vi "JL Dryer Tool.vi"() -> ()   [LabVIEW 2018]
uses:
  GExplorer Support/typedefs/GExplorer_Data_Cluster.ctl
  Common/LabVIEW GEA2 Toolkit/LabVIEW_GEA2_Toolkit.lvlibp/type defs/Data In.ctl
  JL Dryer Tool Support/type defs/ERD_Data_Loop_Control.ctl
  Common/LabVIEW GEA2 Toolkit/LabVIEW_GEA2_Toolkit.lvlibp/type defs/Data Type.ctl
  JL Dryer Tool Support/type defs/ERD_Loop_States_JL.ctl
  Common/LabVIEW GEA2 Toolkit/LabVIEW_GEA2_Toolkit.lvlibp/type defs/ERD Read Data In.ctl
  JL Dryer Tool Support/type defs/Error_Command.ctl
  JL Dryer Tool Support/type defs/DAQ_States.ctl
  JL Dryer Tool Support/type defs/Cont_Send_States.ctl
  <vilib>/DAQmx/write.llb/DAQmx Write (Analog 1D DBL NChan 1Samp).vi
  Common/LabVIEW GEA2 Toolkit/LabVIEW_GEA2_Toolkit.lvlibp/type defs/ERD Write Data In.ctl
  JL Dryer Tool Support/type defs/Flash_Results.ctl
  GEA2 Script/typedefs/Script Info.ctl
  JL Dryer Tool Support/type defs/GEA2_Control_Command.ctl
  JL Dryer Tool Support/type defs/ERD_Loop_Control_Command.ctl
  JL Dryer Tool Support/type defs/DAQ_Control_Command.ctl
  D:/Common/DLLs/GEA3/GeaCommunication.dll
  DLLs/GEA3/GeaCommunication.dll
  Common/LabVIEW GEA2 Toolkit/LabVIEW_GEA2_Toolkit.lvlibp/advanced/GEA2 Message Received Event Handler.vi
  Common/LabVIEW GEA2 Toolkit/LabVIEW_GEA2_Toolkit.lvlibp/advanced/GEA2 Message Sent Event Handler.vi
  Common/LabVIEW GEA2 Toolkit/LabVIEW_GEA2_Toolkit.lvlibp/type defs/Data Out.ctl
  Diagnostics Decode/Type Defs/Diag_FaultTableStatus.ctl
  <vilib>/DAQmx/create/channels.llb/DAQmx Create Channel (DI-Digital Input).vi
  <vilib>/DAQmx/create/channels.llb/DAQmx Create Channel (AO-Voltage-Basic).vi
  <vilib>/DAQmx/create/channels.llb/DAQmx Create Channel (DO-Digital Output).vi
  <vilib>/DAQmx/read.llb/DAQmx Read (Digital 1D Bool NChan 1Samp 1Line).vi
  <vilib>/DAQmx/write.llb/DAQmx Write (Digital 1D Bool NChan 1Samp 1Line).vi
  Common/LabVIEW GEA2 Toolkit/LabVIEW_GEA2_Toolkit.lvlibp/type defs/Source_Destination.ctl
  JL Dryer Tool Support/type defs/ERD_Graph.ctl
  JL Dryer Tool Support/type defs/ERD_Graph_All.ctl
  JL Dryer Tool Support/type defs/Select _Graph_JL.ctl
  JL Dryer Tool Support/type defs/Heat Control.ctl
  JL Dryer Tool Support/type defs/ERD_Always_Show_JL.ctl
  JL Dryer Tool Support/type defs/Programming.ctl
  JL Dryer Tool Support/type defs/Relay_Control.ctl
  JL Dryer Tool Support/type defs/Drum_Light_Control.ctl
  JL Dryer Tool Support/UTL_JL Scaling Factor Folder/Controls/ENUM_JL Scaling Factor_.ctl
  JL Dryer Tool Support/type defs/Cycle Control.ctl
  <vilib>/Platform/fileVersionInfo.llb/FileVersionInformation.ctl
  JL Dryer Tool Support/type defs/Choose_ERD_List.ctl
  Automation/Product Specific/Clothes Care/Justice League/Product Testcode/Diagnostics/TypeDefs/Centauro Diagnostic V3 SnapShot.ctl
  Diagnostics Decode/Type Defs/Diag_FaultSeqEntry.ctl
  Diagnostics Decode/Type Defs/Diag_EntityManifestType.ctl
  Diagnostics Decode/Type Defs/Diag_FaultTableEntry.ctl
  JL Dryer Tool Support/type defs/JL_Diagnost V3 Cycle History.ctl
panel:
  out "Temp ADC":T1
  in  "Read Parametric":bool=TRUE
  in  "Board Index 2":u8 max=0 step=1
  in  "Data ON":bool=TRUE
  out "ERD_Always Show":T2
  in  "Stop":bool
  in  "Reset":bool
  in  "UI Launch":bool
  in  "Tab Control":T3(tab)
  out "Boot Loader Version":T4
  out "UI Version":T5
  out "Version":T6
  in  "Flash Latest":bool
  in  "Filter Data":bool=TRUE
  in  "Start Send":bool
  in  "Ignore this CMD":string
  in  "Msg Rate (ms)":u32=1000 min=50 step=50
  out "Personality Set":u8
  in  "?":u8
  in  "Set Personality":bool
  in  "Programming":T7={"Program"=FALSE, "File Path"=path "", "Program Ind"=FALSE, "Reset Board"=FALSE, "Enter Bootloader"=FALSE, "Result"=9} {"Result" items=["ImageRejected", "BoardNotFound", "UnableToGetGeaConfiguration", "WriteToFlashNotAllowed", "ImageDownloadedSuccessfully", "ImagePresent", "WriteToFlashFailed", "EraseFailed", "CrcFailed", ""]}
  out "CSV File Log Path":path=path "C:/Users/502129737/Desktop/1"
  in  "Clear":bool
  out "GEA2 Log":string
  in  "Board Index":u8 max=10 step=1
  out "Board ID":string="0"
  in  "GEA2 Send":T9={"Source"=228, "Destination"=36, "Command"=0, "Message"=""} {"Command" format="%02x"; "Destination" format="%02x"; "Source" format="%02x"}
  in  "Send Button":bool
  in  "GEA2 Log Length":i32=100000
  in  "Save Log":bool
  in  "#ERDs per message":i32=20
  out "FileVersionInfo":T10
  out "LabView/Version Number":string
  in  "Tool Version":bool=TRUE
  in  "GEA Inputs":T11={"Source"=229, "Destination"=36} {"Destination" format="%.0x"; "Source" format="%.0x"}
  in  "Read ERD List":T12[](array[typedef])=[{"ERD Number"=0, "Data Type"=enum."string"}] {"ERD Number" format="%.0x"}
  out "Read ERD Data Out":cluster{"ERD Number":u16, "Data":string}[](array[cluster]) {"ERD Number" format="%.0x"}
  in  "Read ERD":bool
  in  "Write ERD":bool
  in  "Write ERD List":T14(array[cluster])=[{"ERD Number"=0, "Data Type"=enum."string", "Data"=""}] {"ERD Number" format="%.0x"}
  in  "ERD Graphing ON":bool
  out "ERD Graph  Ind":T15
  in  "ERD Graph Cntrl":T16={"ERD 3"={"ERD #"=61463, "Data Type"=enum."uint16_t", "Scaler"=1}, "ERD 2"={"ERD #"=61461, "Data Type"=enum."uint16_t", "Scaler"=1}, "ERD 1"={"ERD #"=61462, "Data Type"=enum."uint16_t", "Scaler"=1}} {"ERD 1"."Scaler" min=1; "ERD 1"."ERD #" format="%.0x"; "ERD 2"."Scaler" min=1; "ERD 2"."ERD #" format="%.0x"; "ERD 3"."Scaler" min=1; "ERD 3"."ERD #" format="%.0x"}
  in  "Graphing ON":bool=TRUE
  in  "Select Graph":T18
  out "Outlet Thermistor":u16(graph)
  out "Filtered Moisture":u16(graph)
  out "Raw Moisture":u16(graph)
  out "All Loads":u16[][](graph)
  out "ERD 1":dbl(graph)
  out "ERD 2":dbl(graph)
  out "Inlet Thermistor":u16(graph)
  out "ERD 3":dbl(graph)
  in  "Get Faults":bool
  in  "Clear Fault Table Buffer":bool
  in  "Clear Fault Seq Buffer":bool
  out "Fault Sequence Entries":T19[](array[typedef])
  out "Fault Seq Status":T20
  out "Fault Table Entries":T21[](array[typedef])
  out "Fault Table Status":T20
  out "Diagnostic Entity Manifest":T22
  out "Major Version":u8
  out "Minor Version":u8
  out "Fault Set?":bool
  in  "Filter by Count":bool=TRUE
  out "Centauro Fault Snapshot":T23
  in  "Drum Light":T24={"Drum Light ON"=FALSE, "Drum Light OFF"=FALSE, "On Time (s)"=5.0} {"On Time (s)" min=0.0 max=3600.0}
  in  "Relay Control":T25
  in  "LED Control":T26
  in  "Cycle Control":T27
  in  "Enable CC Mode":bool
  in  "Completed Cycles":u16
  in  "Requested Cycles":u16
  in  "TimeBetween Cycles":u32
  in  "Enabled":u8
  in  "ERD Spam GEA Inputs":T11={"Source"=229, "Destination"=36} {"Destination" format="%.0x"; "Source" format="%.0x"}
  in  "Normal Temp V":bool=TRUE
  in  "Manual Inlet":dbl format="%#_13g"
  in  "Manual Outlet":dbl format="%#_13g"
  out "Heat Control":T28
  in  "Init/Scale":T29=enum."Scale Voltage"
  in  "Scalling":T30={"Low  "=1531.0, " High"=6859.0, "Actual Low"=1.0, "Actual High"=4.9}
  in  "Desired FilteredMoisture":dbl=2400.0 min=1000.0 max=6300.0 step=5.0
  out "Drum":bool
  out "Centrifugal Switch":bool caption="Cent SW"
  out "Drum Direction":string
  in  "CentSWControl":bool
  in  "CentSWControlType":bool=TRUE
  out "Steam":bool
  out "Drum Light":bool
  out "Outer Coil":bool
  out "Inner/Gas Coil":bool
  in  "Dither (V)":dbl=0.05 min=0.0 max=1.0 step=0.001 format="%_3g"
  in  "Outlet Therm (F)":dbl(knob)=75.0 min=49.0 max=201.0 step=1.0 scale=50.0..200.0
  in  "Inlet Therm (F)":u16(knob)=75 min=49 max=501 step=1 scale=50.0..500.0
  in  "Moisture (V)":dbl(slide)=1.945 min=0.0 max=5.0 step=0.0001 scale=0.0..5.0 scale format="%#.2f"
  in  "AC Power":bool=TRUE
  in  "Door Status":bool=TRUE
  in  "Start Signal":bool
  out "DAQ Status":string
  in  "Turn On DAQ":bool
  out "DAQ On?":bool
  out "Inlet Voltage":dbl
  out "Outlet Voltage":dbl
  in  "Model":enum16{"Estar Centauro", "GFL"}(ring)
  out "Dampness State":string
  out "Sensor Dry Status":string
  in  "Get Cycle Data":bool
  out "Cycle History Status":T20
  in  "Filter by Status Count":bool=TRUE
  out "JL Cycle History":T31
  in  "Script Log Path":path
  in  "Run Script":bool
  out "Script Pass/Fail?":bool
  out "Script Report Text":string
  in  "stop script":bool
  in  "Script Path":path
  out "Script Info":T32 {"Overall Script File Progress" scale=0.0..1.0; "Elapsed time (s)" format="%#.1f"; "Current Script Progress" scale=0.0..1.0}
  out "Script Error Out":errorcluster
  in  "ERD Read List":T33(array[cluster])=[{"Boolean"=TRUE, "ERD Number"=49, "ERD Name"="Build Number", "Data Type"=enum."uint32_t"}, {"Boolean"=TRUE, "ERD Number"=127, "ERD Name"="Build Hash", "Data Type"=enum."string"}, {"Boolean"=TRUE, "ERD Number"=61467, "ERD Name"="Machine State", "Data Type"=enum."uint8_t"}, {"Boolean"=TRUE, "ERD Number"=61457, "ERD Name"="Relay Status", "Data Type"=enum."string"}, {"Boolean"=TRUE, "ERD Number"=61459, "ERD Name"="Door Switch State", "Data Type"=enum."string"}, {"Boolean"=TRUE, "ERD Number"=61460, "ERD Name"="Door Latch State", "Data Type"=enum."string"}, {"Boolean"=TRUE, "ERD Number"=61461, "ERD Name"="Inlet Thermistor", "Data Type"=enum."uint16_t"}, {"Boolean"=TRUE, "ERD Number"=61462, "ERD Name"="Outlet Thermistor", "Data Type"=enum."uint16_t"}, {"Boolean"=TRUE, "ERD Number"=61468, "ERD Name"="Control Lock State", "Data Type"=enum."string"}, {"Boolean"=TRUE, "ERD Number"=61483, "ERD Name"="Signal Volume", "Data Type"=enum."string"}, {"Boolean"=TRUE, "ERD Number"=61582, "ERD Name"="Drum Light", "Data Type"=enum."string"}, {"Boolean"=TRUE, "ERD Number"=61478, "ERD Name"="Delay Time", "Data Type"=enum."string"}, {"Boolean"=TRUE, "ERD Number"=8275, "ERD Name"="Ext. Tumble", "Data Type"=enum."string"}, {"Boolean"=TRUE, "ERD Number"=8272, "ERD Name"="Temp Level", "Data Type"=enum."string"}, {"Boolean"=TRUE, "ERD Number"=8269, "ERD Name"="Dryness Level", "Data Type"=enum."string"}, {"Boolean"=TRUE, "ERD Number"=8262, "ERD Name"="eDry", "Data Type"=enum."string"}, {"Boolean"=TRUE, "ERD Number"=61495, "ERD Name"="Time Level", "Data Type"=enum."string"}, {"Boolean"=TRUE, "ERD Number"=8266, "ERD Name"="Damp Alert", "Data Type"=enum."string"}, {"Boolean"=TRUE, "ERD Number"=61501, "ERD Name"="Detangle", "Data Type"=enum."string"}, {"Boolean"=TRUE, "ERD Number"=61510, "ERD Name"="MyCycle", "Data Type"=enum."string"}, {"Boolean"=TRUE, "ERD Number"=61594, "ERD Name"="Cycle Engine State", "Data Type"=enum."string"}, {"Boolean"=TRUE, "ERD Number"=61597, "ERD Name"="Cycle Selected", "Data Type"=enum."string"}, {"Boolean"=TRUE, "ERD Number"=61443, "ERD Name"="Tune ID", "Data Type"=enum."string"}, {"Boolean"=TRUE, "ERD Number"=61503, "ERD Name"="Delay Option", "Data Type"=enum."string"}, {"Boolean"=TRUE, "ERD Number"=61619, "ERD Name"="Restriction Detection Status", "Data Type"=enum."string"}, {"Boolean"=TRUE, "ERD Number"=61618, "ERD Name"="Vent Restriction", "Data Type"=enum."string"}, {"Boolean"=TRUE, "ERD Number"=61611, "ERD Name"="Load Size By Contact", "Data Type"=enum."string"}, {"Boolean"=TRUE, "ERD Number"=61613, "ERD Name"="Load Size by Temp", "Data Type"=enum."string"}, {"Boolean"=TRUE, "ERD Number"=61615, "ERD Name"="LoadSizeByAggregation", "Data Type"=enum."string"}, {"Boolean"=TRUE, "ERD Number"=61605, "ERD Name"="Sensor Dry Status", "Data Type"=enum."string"}, {"Boolean"=TRUE, "ERD Number"=61626, "ERD Name"="Check Dampness State", "Data Type"=enum."string"}, {"Boolean"=TRUE, "ERD Number"=61624, "ERD Name"="MoistureSensorRawAdcFromMc", "Data Type"=enum."string"}, {"Boolean"=TRUE, "ERD Number"=62242, "ERD Name"="SmoothMoistureReading", "Data Type"=enum."string"}, {"Boolean"=TRUE, "ERD Number"=61463, "ERD Name"="Filtered Moisture", "Data Type"=enum."string"}, {"Boolean"=TRUE, "ERD Number"=61608, "ERD Name"="TargetMoistureVoltage", "Data Type"=enum."string"}, {"Boolean"=TRUE, "ERD Number"=61609, "ERD Name"="TargetMoistureVoltageReached", "Data Type"=enum."string"}, {"Boolean"=TRUE, "ERD Number"=61719, "ERD Name"="MaxFilteredMoistureVoltageDuringASensingCycle", "Data Type"=enum."string"}, {"Boolean"=TRUE, "ERD Number"=61555, "ERD Name"="TrimmerBothCoilInhibitRequest", "Data Type"=enum."string"}, {"Boolean"=TRUE, "ERD Number"=61567, "ERD Name"="TrimmerInhibitRelay1", "Data Type"=enum."string"}, {"Boolean"=TRUE, "ERD Number"=61568, "ERD Name"="TrimmerInhibitRelay2", "Data Type"=enum."string"}, {"Boolean"=TRUE, "ERD Number"=61549, "ERD Name"="HeatControlParametricData", "Data Type"=enum."string"}, {"Boolean"=TRUE, "ERD Number"=61610, "ERD Name"="EOC Reason", "Data Type"=enum."string"}, {"Boolean"=TRUE, "ERD Number"=61600, "ERD Name"="Heat Control Request", "Data Type"=enum."string"}, {"Boolean"=TRUE, "ERD Number"=61677, "ERD Name"="CoolDownStepStatus", "Data Type"=enum."string"}, {"Boolean"=TRUE, "ERD Number"=61554, "ERD Name"="OverTempHeaterInhibitRequest", "Data Type"=enum."string"}, {"Boolean"=TRUE, "ERD Number"=61565, "ERD Name"="EcoDryInhibitRelay1", "Data Type"=enum."string"}, {"Boolean"=TRUE, "ERD Number"=61566, "ERD Name"="EcoDryInhibitRelay2", "Data Type"=enum."string"}, {"Boolean"=TRUE, "ERD Number"=61743, "ERD Name"="ReverseDrumInhibitRelay1", "Data Type"=enum."string"}, {"Boolean"=TRUE, "ERD Number"=61744, "ERD Name"="ReverseDrumInhibitRelay2", "Data Type"=enum."string"}, {"Boolean"=TRUE, "ERD Number"=61556, "ERD Name"="NormalHeatControlMethodStatus", "Data Type"=enum."string"}, {"Boolean"=TRUE, "ERD Number"=61557, "ERD Name"="FallbackHeatControlMethodStatus", "Data Type"=enum."string"}, {"Boolean"=TRUE, "ERD Number"=61479, "ERD Name"="Remaining Cycle Time", "Data Type"=enum."string"}, {"Boolean"=TRUE, "ERD Number"=61698, "ERD Name"="InitialHeatingCycleTimeSeconds", "Data Type"=enum."string"}, {"Boolean"=TRUE, "ERD Number"=62214, "ERD Name"="InletTemperatureRawAdc\n", "Data Type"=enum."string"}, {"Boolean"=TRUE, "ERD Number"=62215, "ERD Name"="OutletTemperatureRawAdc", "Data Type"=enum."string"}, {"Boolean"=TRUE, "ERD Number"=61607, "ERD Name"="SensingCycleTotalDryingTimeSeconds", "Data Type"=enum."string"}, {"Boolean"=TRUE, "ERD Number"=61563, "ERD Name"="TimedCycleTotalDryingTimeSeconds", "Data Type"=enum."string"}, {"Boolean"=TRUE, "ERD Number"=61628, "ERD Name"="TimeToReachTargetVoltageSeconds", "Data Type"=enum."string"}, {"Boolean"=TRUE, "ERD Number"=61617, "ERD Name"="Dry Load Detection", "Data Type"=enum."string"}, {"Boolean"=TRUE, "ERD Number"=63510, "ERD Name"="Sensor DryTemp Multiplier 100", "Data Type"=enum."string"}, {"Boolean"=TRUE, "ERD Number"=61728, "ERD Name"="Erd_EcoDrySensorDryProfileSelectorStatus", "Data Type"=enum."string"}, {"Boolean"=TRUE, "ERD Number"=61729, "ERD Name"="Erd_EcoDrySensorDryProfileSelectorResultmeInSeconds", "Data Type"=enum."string"}, {"Boolean"=TRUE, "ERD Number"=61736, "ERD Name"="Erd_EcoDryControllerStatus", "Data Type"=enum."string"}, {"Boolean"=TRUE, "ERD Number"=61737, "ERD Name"="Erd_EcoDryRelay1TimerData", "Data Type"=enum."string"}, {"Boolean"=TRUE, "ERD Number"=61738, "ERD Name"="Erd_EcoDryRelay2TimerData", "Data Type"=enum."string"}, {"Boolean"=TRUE, "ERD Number"=61739, "ERD Name"="Erd_EcoDryStage2TransitionTimeInSeconds", "Data Type"=enum."string"}, {"Boolean"=TRUE, "ERD Number"=8193, "ERD Name"="Erd_MachineSubCycle", "Data Type"=enum."string"}, {"Boolean"=TRUE, "ERD Number"=61606, "ERD Name"="Erd_ElapsedCycleTimeSeconds2TransitionTimeInSeconds", "Data Type"=enum."string"}, {"Boolean"=TRUE, "ERD Number"=63489, "ERD Name"="SensorDryDampSmallRestrictionSmallLoad\natus", "Data Type"=enum."string"}] {"ERD Number" format="%.0x"}
  in  "Load ERD List":T34=enum."QA ERDs"
  out "Error Out":errorcluster
  in  "Error In":errorcluster
  # "The higher this number is the less reliable the bus becomes.\nLower will increase the delay for the ERD Array to populate.\nNo greater than 30 per msg is recommended. (crashing can occur)"
  # "Software Version"
  # "Critical Version"
  # "Non-Critical"
  # "Software Version"
  # "Critical Version"
  # "Non-Critical"
  # "XML Crit Ver"
  # "XML Non-Crit"
  # "Build Number"
  # "Build Hash"
  # "Personality"
  # "ERD_Graph_All.ctlERD_Graph_All.ctlMust input av valid ERD# and Data Type DO NOT Leave Blank If no scaler use value of 01"
  # "This controls destination of ERD Spam.\nYou should never change source unless\nyou want to see the spam in the GEA log."
  # "Continuous cycle Config"
  # "Filtered Moisture"
  # "Voltage (DAQ)"
  # "Measured Range"
  # "Centrifugal Switch"
  # "On"
  # "Normal"
  # "Off"
  # "Manual"
  # "Insert all New ERDs above F801..ensure this is the last ERD in the list"
  # "Contact:\n\nTerrance Bradford\nTerrance.Bradford@geappliances.com"
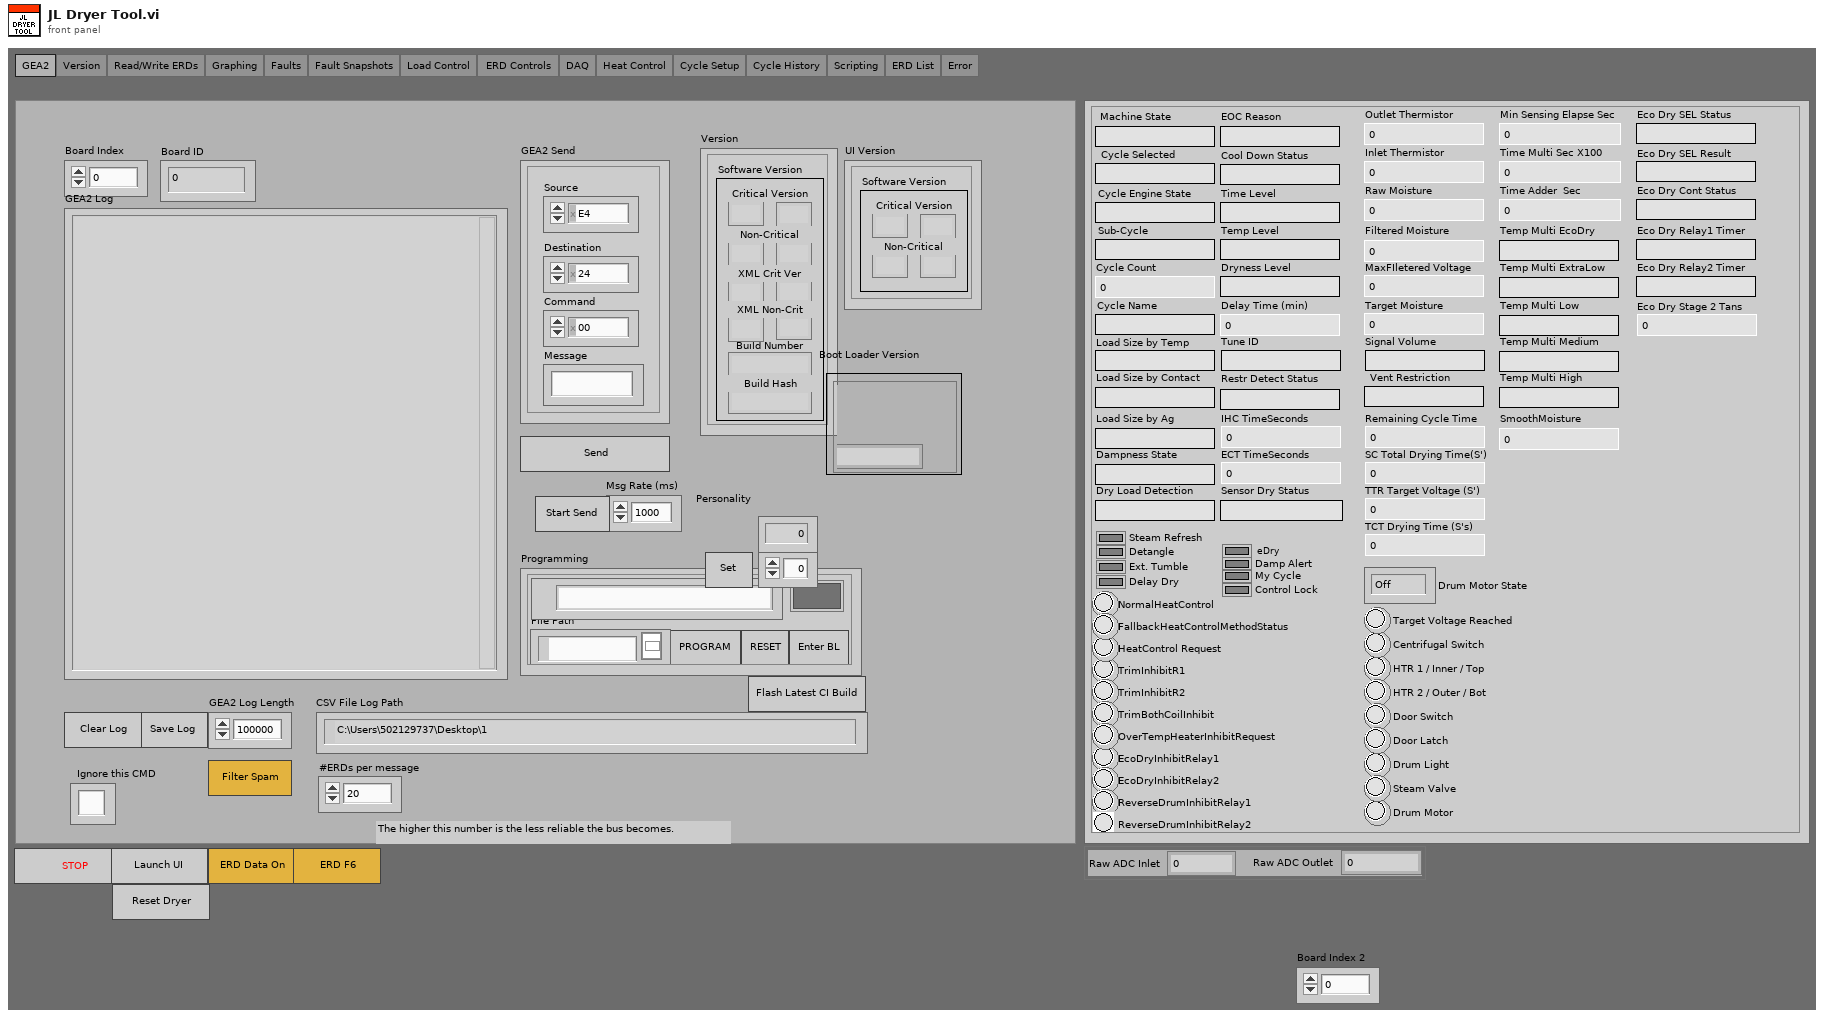
[diagram p1: front panel]
types:
  T1 = cluster{"Raw ADC Outlet":u16, "Raw ADC Inlet":u16}
  T2 = typedef "ERD_Always_Show_JL.ctl" = cluster{"Inlet Thermistor":u16, "Machine State":string, "Filtered Moisture":u16, "Cycle Selected":string, "HTR 1 / Inner / Top":bool, "HTR 2 / Outer / Bot":bool, "Door Switch":bool, "Drum Light":bool, "Cycle Engine State":string, "Centrifugal Switch":bool, "Drum Motor":bool, "Cycle Count":u32, "Ext. Tumble":bool, "eDry":bool, "Temp Level":string, "Dryness Level":string, "Time Level":string, "Delay Time (min)":u16, "Steam Refresh":bool, "Damp Alert":bool, "Sub-Cycle":string, "Outlet Thermistor":u16, "Target Moisture":u16, "Remaining Cycle Time":u32, "Raw Moisture":u16, "Cycle Name":string, "My Cycle":bool, "Delay Dry":bool, "Detangle":bool, "Control Lock":bool, "Steam Valve":bool, "Door Latch":bool, "Signal Volume":string, "Tune ID":string, "Restr Detect Status":string, "Vent Restriction":string, "Load Size by Contact":string, "Load Size by Temp":string, "EOC Reason":string, "Sensor Dry Status":string, "Dampness State":string, "Target Voltage Reached":bool, "TrimInhibitR1":bool, "TrimInhibitR2":bool, "TrimBothCoilInhibit":bool, "NormalHeatControl":bool, "HeatControl Request":bool, "Cool Down Status":string, "EcoDryInhibitRelay1":bool, "EcoDryInhibitRelay2":bool, "ReverseDrumInhibitRelay1":bool, "ReverseDrumInhibitRelay2":bool, "OverTempHeaterInhibitRequest":bool, "FallbackHeatControlMethodStatus":bool, "IHC TimeSeconds":u32, "ECT TimeSeconds ":u32, "SC Total Drying Time(S')":u32, "TTR Target Voltage (S')":u32, "TCT Drying Time (S's)":u32, "Drum Motor State":enum16{"Off", "Cw", "Ccw", "Max"}, "Load Size by Ag":string, "MaxFIletered Voltage":u16, "Dry Load Detection":string, "Min Sensing Elapse Sec":u32, "Time Multi Sec X100":u32, "Time Adder  Sec":u32, "Temp Multi EcoDry":string, "Temp Multi ExtraLow":string, "Temp Multi Low ":string, "Temp Multi Medium":string, "Temp Multi High":string, "SmoothMoisture":u16, "Eco Dry SEL Status":string, "Eco Dry SEL Result":string, "Eco Dry Cont Status":string, "Eco Dry Relay1 Timer":string, "Eco Dry Relay2 Timer ":string, "Eco Dry Stage 2 Tans ":u32}
  T3 = enum32{"GEA2", "Version", "Read/Write ERDs", "Graphing", "Faults", "Fault Snapshots", "Load Control", "ERD Controls ", "DAQ", "Heat Control", "Cycle Setup", "Cycle History", "Scripting", "ERD List", "Error"}
  T4 = cluster{"UI BL Version":string, "MC BL Version":string}
  T5 = cluster{"Critical Major":string, "Critical Minor":string, "Non-Critical Minor":string, "Non-Critical Major":string}
  T6 = cluster{"Critical Major":string, "Critical Minor":string, "Non-Critical Minor":string, "Non-Critical Major":string, "XML Crit Minor":string, "XMLCrit Major":string, "Build Number":string, "XML Non-crit Minor":string, "Xml Non-crit Major":string, "Build Hash":string}
  T7 = typedef "Programming.ctl" = cluster{"Program":bool, "File Path":path, "Program Ind":bool, "Reset Board":bool, "Enter Bootloader":bool, "Result":T8}
  T8 = typedef "Flash_Results.ctl" = i32
  T9 = typedef "LabVIEW_GEA2_Toolkit.lvlibp/Data In.ctl" = cluster{"Source":u8, "Destination":u8, "Command":u8, "Message":string}
  T10 = typedef "FileVersionInformation.ctl" = cluster{"FileVersion":string, "ProductName":string, "InternalName":string, "CompanyName":string, "LegalCopyright":string, "FileDescription":string}
  T11 = typedef "LabVIEW_GEA2_Toolkit.lvlibp/Source_Destination.ctl" = cluster{"Source":u8, "Destination":u8}
  T12 = typedef "LabVIEW_GEA2_Toolkit.lvlibp/ERD Read Data In.ctl" = cluster{"ERD Number":u16, "Data Type":T13}
  T13 = typedef "LabVIEW_GEA2_Toolkit.lvlibp/Data Type.ctl" = enum16{"string", "boolean", "uint8_t", "uint16_t", "uint32_t", "uint64_t", "int8_t", "int16_t", "int32_t", "int64_t"}
  T14 = cluster{"ERD Number":u16, "Data Type":T13, "Data":string}[]
  T15 = cluster{"ERD Value 1":dbl, "ERD Value 2":dbl, "ERD Value 3":dbl}
  T16 = typedef "ERD_Graph_All.ctl" = cluster{"ERD 3":T17, "ERD 2":T17, "ERD 1":T17}
  T17 = typedef "ERD_Graph.ctl" = cluster{"ERD #":u16, "Data Type":T13, "Scaler":u32}
  T18 = typedef "Select _Graph_JL.ctl" = enum16{"All Loads", "Inlet Thermistor", "Outlet Thermistor", "Raw Moisture", "Filtered Moisture", "ERD 1", "ERD 2", "ERD 3"}
  T19 = typedef "Diag_FaultSeqEntry.ctl" = cluster{"Cycle #":u32, "Time":u32, "F Code":string, "F Active":bool}
  T20 = typedef "Diag_FaultTableStatus.ctl" = cluster{"Cur Index":u16, "Count":u16, "Ov Cnt":u16}
  T21 = typedef "Diag_FaultTableEntry.ctl" = cluster{"Cycle #":u32, "Time":u32, "F Code":string, "F Count":u16, "F Active":bool}
  T22 = typedef "Diag_EntityManifestType.ctl" = cluster{"ID":u8, "Data Ver Maj":u8, "Data Ver Min":u8, "Fault Table?":bool, "Fault Table Snap?":bool, "Fault Seq?":bool, "Fault Seq Snap?":bool, "Cycle History Seq?":bool, "Fault Table Entry Count":u16, "Fault Seq Entry Count":u16, "Cycle History Entry Count":u16, "Cycle Count":u32, "Entity Run Time (Min)":u32}
  T23 = typedef "Centauro Diagnostic V3 SnapShot.ctl" = string[][]
  T24 = typedef "Drum_Light_Control.ctl" = cluster{"Drum Light ON":bool, "Drum Light OFF":bool, "On Time (s)":dbl}
  T25 = typedef "Relay_Control.ctl" = cluster{"Drum Motor":bool, "HTR 2 / Outer / Bot":bool, "Steam Valve":bool, "Relays ON":bool, "Relays OFF":bool, "HTR 1 / Inner / Top":bool}
  T26 = cluster{"ALL LEDs ON":bool, "ALL LEDs OFF":bool, "Reset LEDs":bool}
  T27 = typedef "Cycle Control.ctl" = cluster{"Start Cycle":bool, "Cycle Selection":u8, "Stop Cycle":bool, "Pause Cycle":bool, "Resume Cycle":bool, "Select Cycle":bool}
  T28 = typedef "Heat Control.ctl" = cluster{"Htr1 InletLowLim":string, "Htr1 InletUpLim":string, "Htr1 OutletLowLim":string, "Htr1 OutletUpLim":string, "Htr1 FallBackON(s)":string, "Htr1 FallBackOFF(s)":string, "Htr1":bool, "Htr2 InletLowLim":string, "Htr2 InletUpLim":string, "Htr2 OutletLowLim":string, "Htr2 OutletUpLim":string, "Htr2 FallBackON(s)":string, "Htr2 FallBackOFF(s)":string, "Htr2":bool}
  T29 = typedef "ENUM_JL Scaling Factor_.ctl" = enum16{"Init", "Scale Voltage", "Flush Slope"}
  T30 = cluster{"Low  ":dbl, " High":dbl, "Actual Low":dbl, "Actual High":dbl}
  T31 = typedef "JL_Diagnost V3 Cycle History.ctl" = string[][]
  T32 = typedef "Script Info.ctl" = cluster{"Overall Script File Progress":dbl, "Current Script Progress":dbl, "Script":string, "Test":string, "Elapsed time (s)":dbl, "Done?":bool}
  T33 = cluster{"Boolean":bool, "ERD Number":u16, "ERD Name":string, "Data Type":enum16{"string", "boolean", "uint8_t", "uint16_t", "uint32_t", "uint64_t", "int8_t", "int16_t", "int32_t", "int64_t"}}[]
  T34 = typedef "Choose_ERD_List.ctl" = enum16{"Base ERDs", "QA ERDs", "MABE ERD List", "EcoDry Evaluation ERD List", "ClothDampnessCheck ERD List"}
  T35 = typedef "Cont_Send_States.ctl" = enum16{"Run", "Shutdown"}
  T36 = typedef "DAQ_States.ctl" = enum16{"Wait for Init", "Rename Devices", "Verify Hardware", "Initialize", "Run", "Shutdown", "Exit"}
  T37 = typedef "ERD_Data_Loop_Control.ctl" = cluster{"Data":variant, "State":T38}
  T38 = typedef "ERD_Loop_States_JL.ctl" = enum16{"Init", "Build ERD Read List", "Read ERDs", "Get Version", "Check Load Size", "Update UI", "Update Graphs", "Read Faults", "Log Data", "Pause", "Shutdown"}
  T39 = typedef "Error_Command.ctl" = enum16{"Initialize", "Handle Errors", "Report Errors"}
  T40 = typedef "GExplorer_Data_Cluster.ctl" = cluster{"Data":variant, "State":enum16{"Add to Log", "Clear", "Shutdown"}}
  T41 = enum8{"Enabled", "Disabled", "Disabled and Grayed Out"}
  T42 = typedef "LabVIEW_GEA2_Toolkit.lvlibp/ERD Write Data In.ctl" = cluster{"ERD Number":u16, "Data Type":T13, "Data":string}
  T43 = enum16{"UI Application APL", "UI Parametric APL", "MC APL"}
  T44 = typedef "GEA2_Control_Command.ctl" = enum16{"Initialize", "Shutdown"}
  T45 = typedef "ERD_Loop_Control_Command.ctl" = enum16{"Initialize", "Shutdown"}
  T46 = typedef "DAQ_Control_Command.ctl" = enum16{"Initialize", "Shutdown", "Exit"}
  T47 = typedef "LabVIEW_GEA2_Toolkit.lvlibp/Data Out.ctl" = cluster{"Source":u8, "Destination":u8, "Command":u8, "Length":u8, "CRC":u16, "Message":string}
  T48 = typedef "LabVIEW_GEA2_Toolkit.lvlibp/ERD Read Data Out.ctl" = cluster{"ERD Number":u16, "Data":string}
  T49 = typedef "All_Bundled_Data_JL.ctl" = cluster{"Version":T50, "ERD_Always Show":T2, "Personality Set":u8, "CSV File String Arrays":T51, "Fault Table Array ":T52, "Heat Control":T28, "Temp ADC":cluster{"Raw ADC Outlet":u16, "Raw ADC Inlet":u16}, "UI Version":cluster{"Critical Major":string, "Critical Minor":string, "Non-Critical Minor":string, "Non-Critical Major":string}, "Boot Loader Version":cluster{"UI BL Version":string, "MC BL Version":string}}
  T50 = typedef "Version.ctl" = cluster{"Critical Major":string, "Critical Minor":string, "Non-Critical Minor":string, "Non-Critical Major":string, "XML Crit Minor":string, "XMLCrit Major":string, "Build Number":string, "XML Non-crit Minor":string, "Xml Non-crit Major":string, "Build Hash":string}
  T51 = typedef "CSV_File_String_Arrays.ctl" = cluster{"ERD Number Array":string[], "ERD Name Array":string[], "ERD Converted String Data":string[]}
  T52 = typedef "Fault Table Array.ctl" = T53[]
  T53 = typedef "Fault_Table_Info.ctl" = cluster{"Cycle Count":u32, " Runtime (min) ":u32, "Fault Status":string, "Fault ID":string, "Fault Count":u16}
  T54 = typedef "F6_ERD_Control.ctl" = cluster{"EcoDryEnabledFlag":string, "KeyCycleId":u8, "CycleType":string, "Time LVL option 5":u32, "Time LVL option 4":u32, "Time LVL option _3":u32, "Time LVL option _2":u32, "Time LVL option _1":u32, "Time LVL option _0":u32, "CoolDownTimeInSeconds":u32, "TimeAdjustTimeCycleMinimumTimeInSeconds":u32, "TimeAdjustTimeCycleMaximumTimeInSeconds":u32, "TimeAdjustTimeCycleStandardAdjustTimeInSeconds":u32, "TimeAdjustTimeCycleSlewAdjustTimeInSeconds":u32, "ExtendedTumbleTimeInSeconds":u32, "SanitizeMaxDryTimeInSeconds":u32, "TemperatureDefault Level":u8, "Temperature ecoDryDefualtLevel":u8, "DrynessDefault Level":u8, "DrynessDefault ecoDryDefualtLevel":u8, "TimeAdjust defaultLevel":u8, "TimeAdjust ecoDryDefualtLevel":u8, "TimeLevelDefault Level":u8, "TimeLevelDefault Eco Dry":u8, "EStarSensorDry Default Level":u8, "EStarSensorDry ecoDryDefaultLevel":u8, "EcoDryDefault Level":u8, "EcoDryDefault EcoDryDefaultLevel ":u8, "ExtendedTumble Default Level":u8, "ExtendedTumble  EcoDryDefaultLevel":u8, "Sanitize Default Level":u8, "Sanitize ecoDryDefualtLevel":u8, "MyCycleDefault Level":u8, "MyCycleDefault ecoDryDefualtLevel":u8, "StartPause Default Level":u8, "StartPause ecoDryDefualtLevel":u8, "Power Default Level":u8, "Power ecoDryDefualtLevel":u8, "KeyVolume Default Level":u8, "KeyVolume ecoDryDefualtLevel":u8, "AlertVolume Default Level":u8, "AlertVolume ecoDryDefualtLevel":u8, "ControlLock Default Level":u8, "ControlLock EecoDryDefualtLevel":u8, "HeatControlRelay1EcoDryParametricDataEntry\nHeatControlTemperatureLimit_InletLower":u16, "HeatControlRelay1EcoDryParametricDataEntry\nHeatControlTemperatureLimit_InletUpper":u16, "HeatControlRelay1EcoDryParametricDataEntry\nHeatControlTemperatureLimit_OutletLower":u16, "HeatControlRelay1EcoDryParametricDataEntry\nHeatControlTemperatureLimit_OutletUpper":u16, "HeatControlRelay1EcoDryParametricDataEntry\nonTimeInSeconds":u8, "HeatControlRelay1EcoDryParametricDataEntry\noffTimeInSeconds":u8, "HeatControlRelay1EcoDryParametric\nDataEntryChange ":bool, "HeatControlRelay2 EcoDryParametricDataEntry\nHeatControlTemperatureLimit_InletLower":u16, "HeatControlRelay2 EcoDryParametricDataEntry\nHeatControlTemperatureLimit_InletUpper ":u16, "HeatControlRelay2EcoDryParametricDataEntry\nHeatControlTemperatureLimit_OutletLower ":u16, "HeatControlRelay2EcoDryParametricDataEntry\nHeatControlTemperatureLimit_OutletUpper":u16, "HeatControlRelay2EcoDryParametricDataEntry\nonTimeInSeconds ":u8, "HeatControlRelay2EcoDryParametricDataEntry\noffTimeInSeconds ":u8, "HeatControlRelay2EcoDry\nParametricDataEntryChange":bool, "DampAlert Default Level":u8, "DampAlert ecoDryDefaultLevel":u8, "Detangle Default Level ":u8, "Detangle ecoDryDefaultLevel":u8, "DelayStart Default Level":u8, "DelayStart ecoDryDefaultLevel":u8, "CycleAllowsInventoryChangeChange":bool, "TemperatureAllowable":u8, "DrynessAllowable":u8, "TimeLevelAllowable":u8, "EcoDryAllowable":u8, "ExtendedTumbleAllowable":u8, "DampAlertAllowable":u8, "DetangleAllowable":u8, "DelayStartAllowable":u8, "SanitizeAllowable":u8, "MyCycleAllowable":u8, "TimeAdjustAllowable":u8, "Power Allowable":u8, "KeyVolumeAllowable":u8, "AlertVolumeAllowable":u8, "ControlLockAllowable":u8, "EStarSensorDryAllowable":string, "StartPauseAllowable":u8, "EcoDryStage1Heater2\nActiveSeconds":u32, "EcoDryStage2PeriodSeconds":u32, "EcoDryStage2Heater1\nActiveSeconds":u32, "EcoDryStage2Heater2\nActiveSeconds":u32, "EcoDryStage1Heater1\nActiveSeconds":u32, "EcoDryStage1PeriodSeconds":u32, "EcoDryStage2DurationSeconds":u32, "CoolDownAdaptiveTargetTemperature":u16}
  T55 = enum32{"invalid app kind", "Development System", "Run Time System", "Student Edition", "Embedded LabVIEW", "Evaluation", "Custom"}
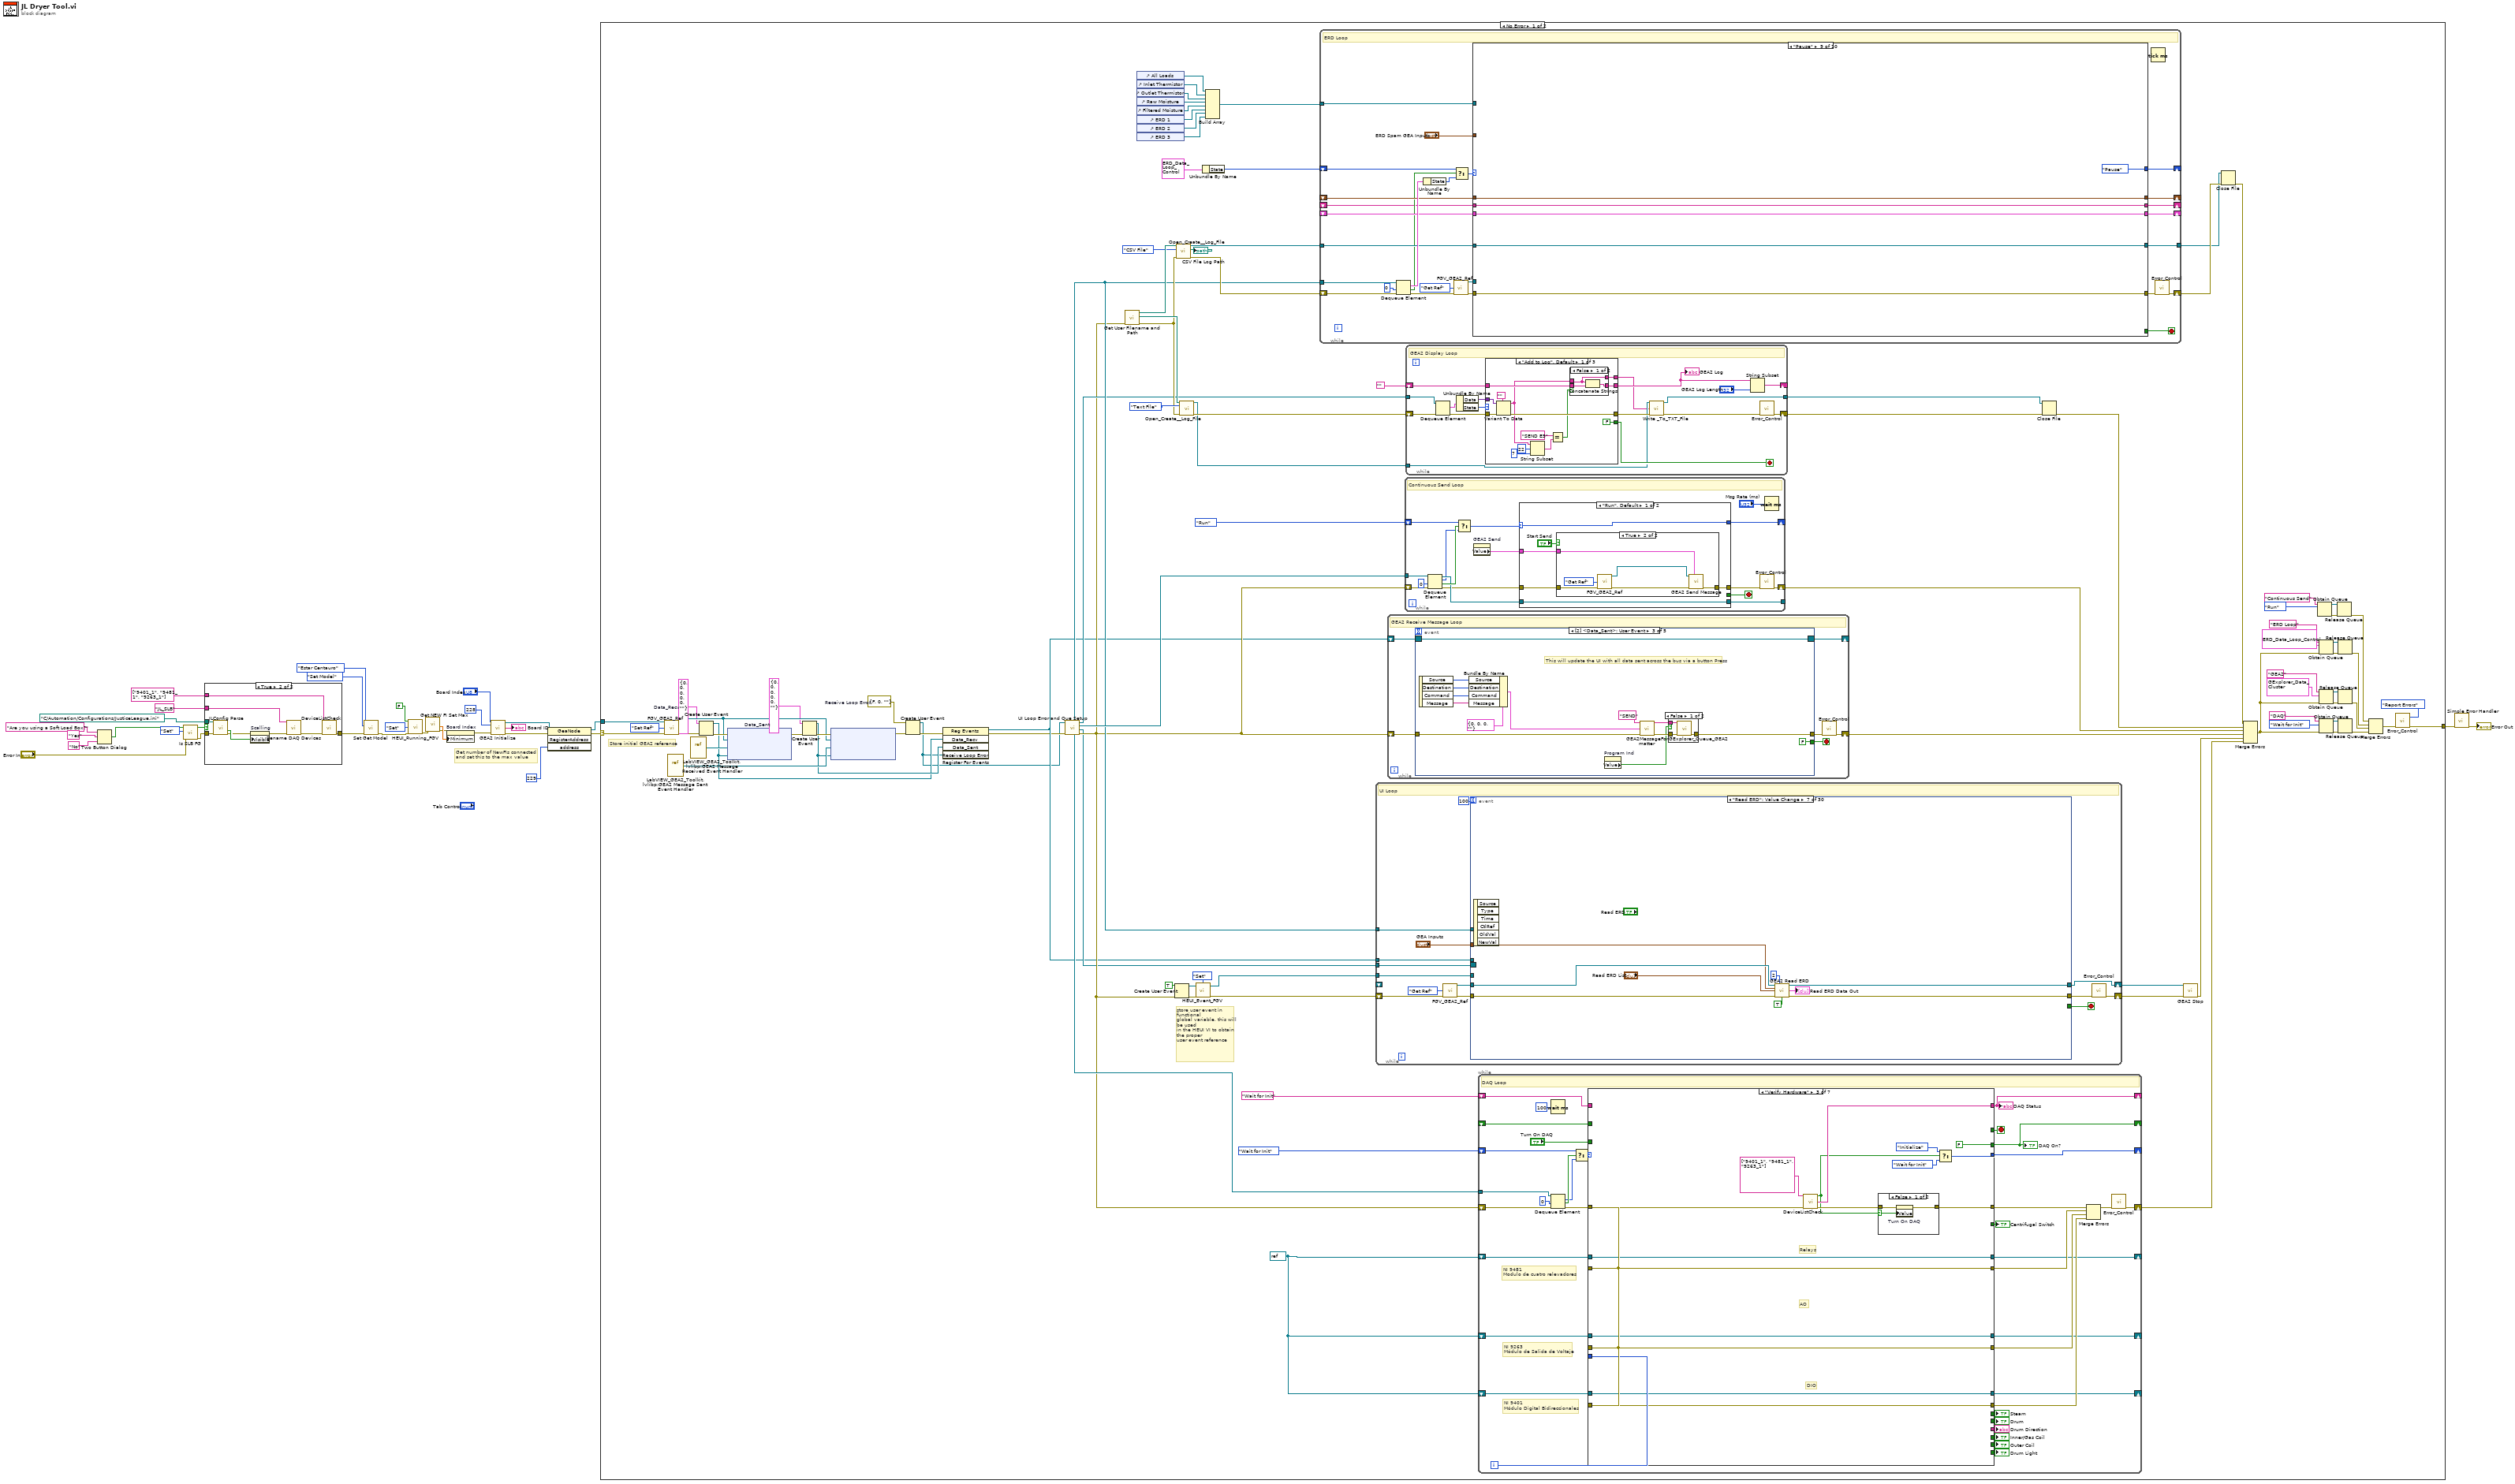
[diagram p0: block diagram]
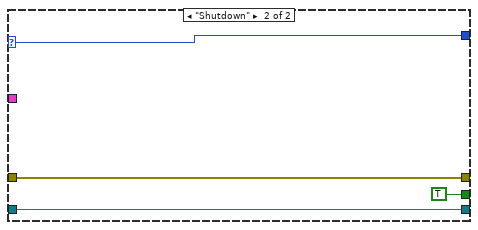
[diagram p4: hidden frame]
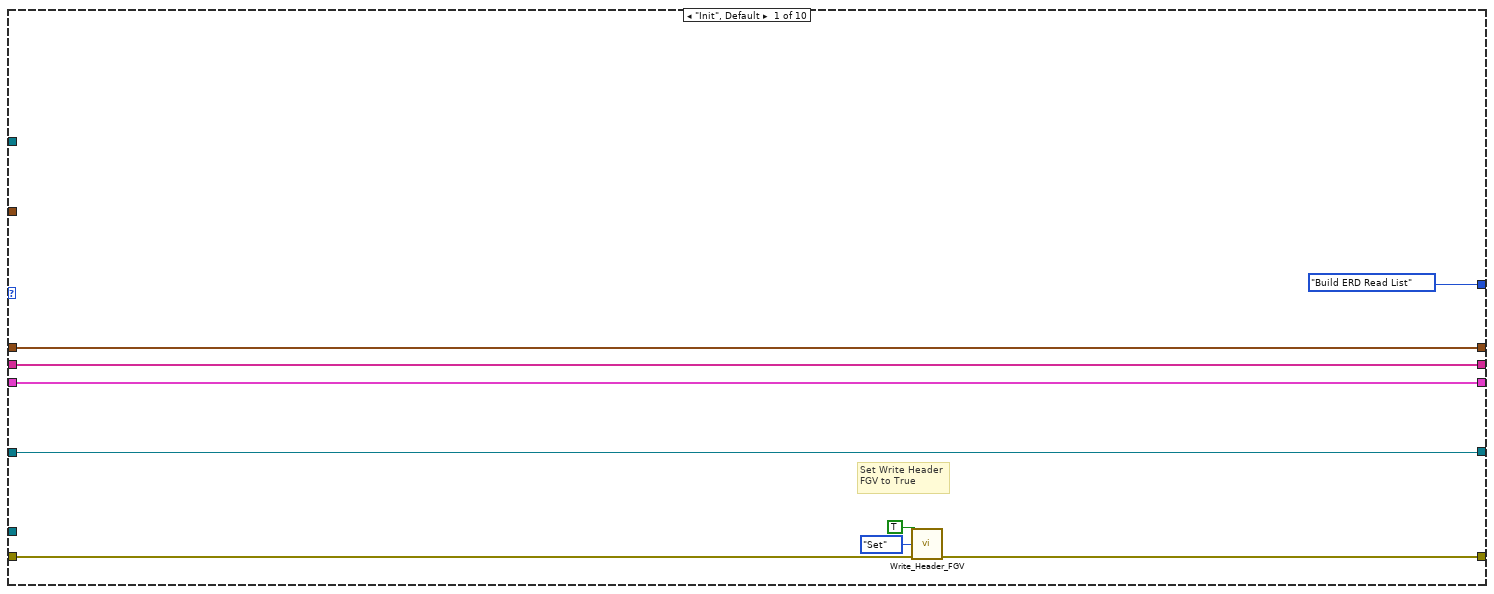
[diagram p5: hidden frame]
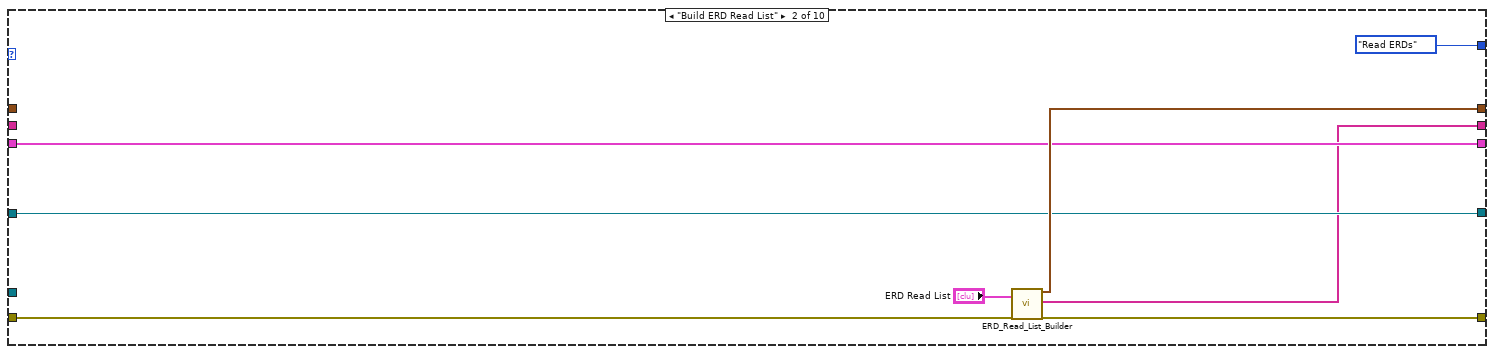
[diagram p6: hidden frame]
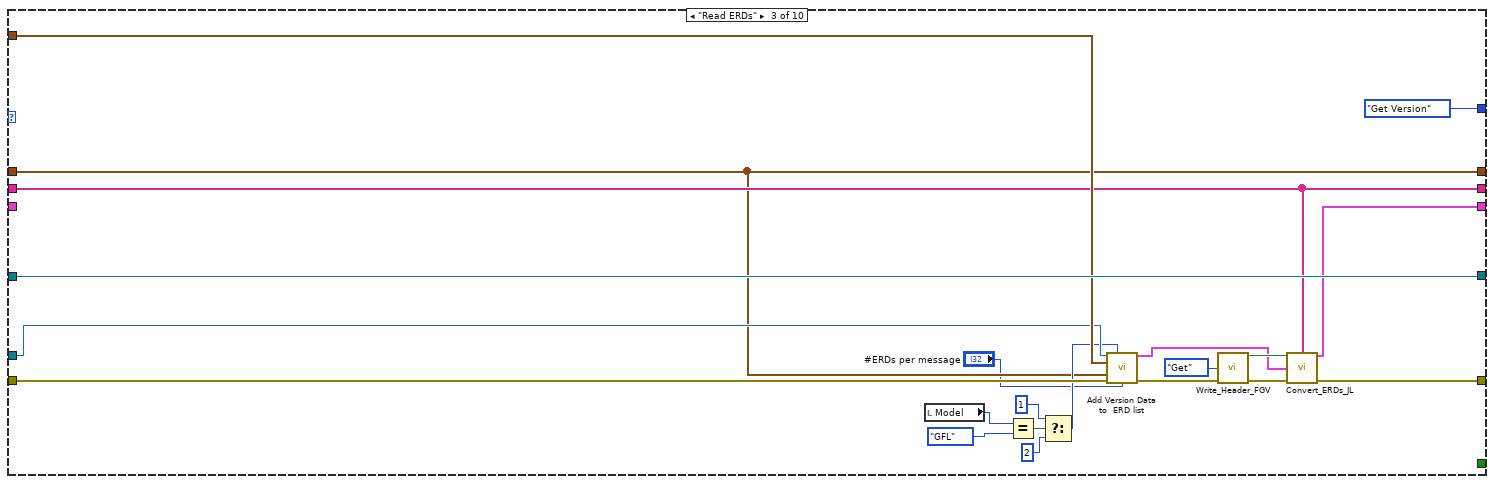
[diagram p7: hidden frame]
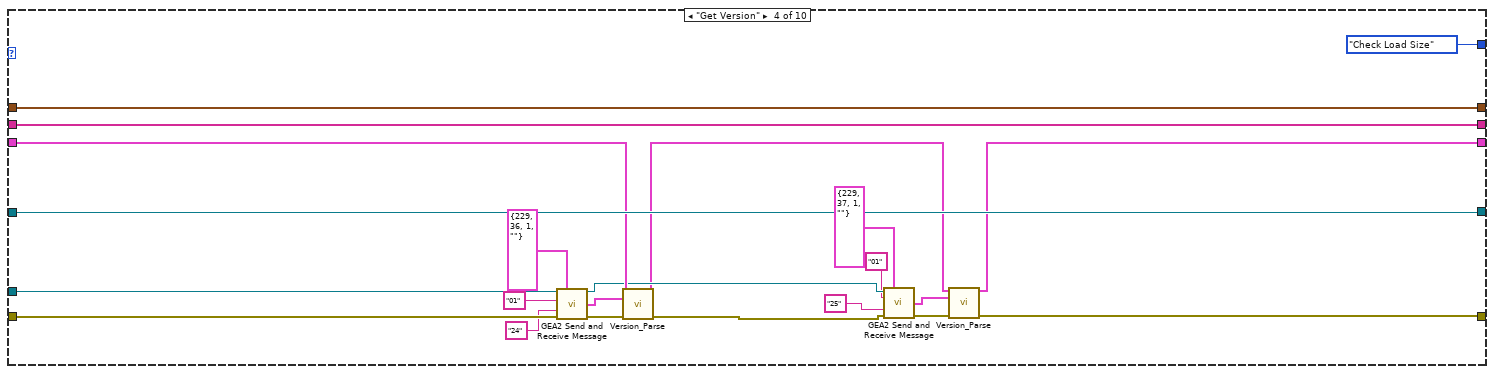
[diagram p8: hidden frame]
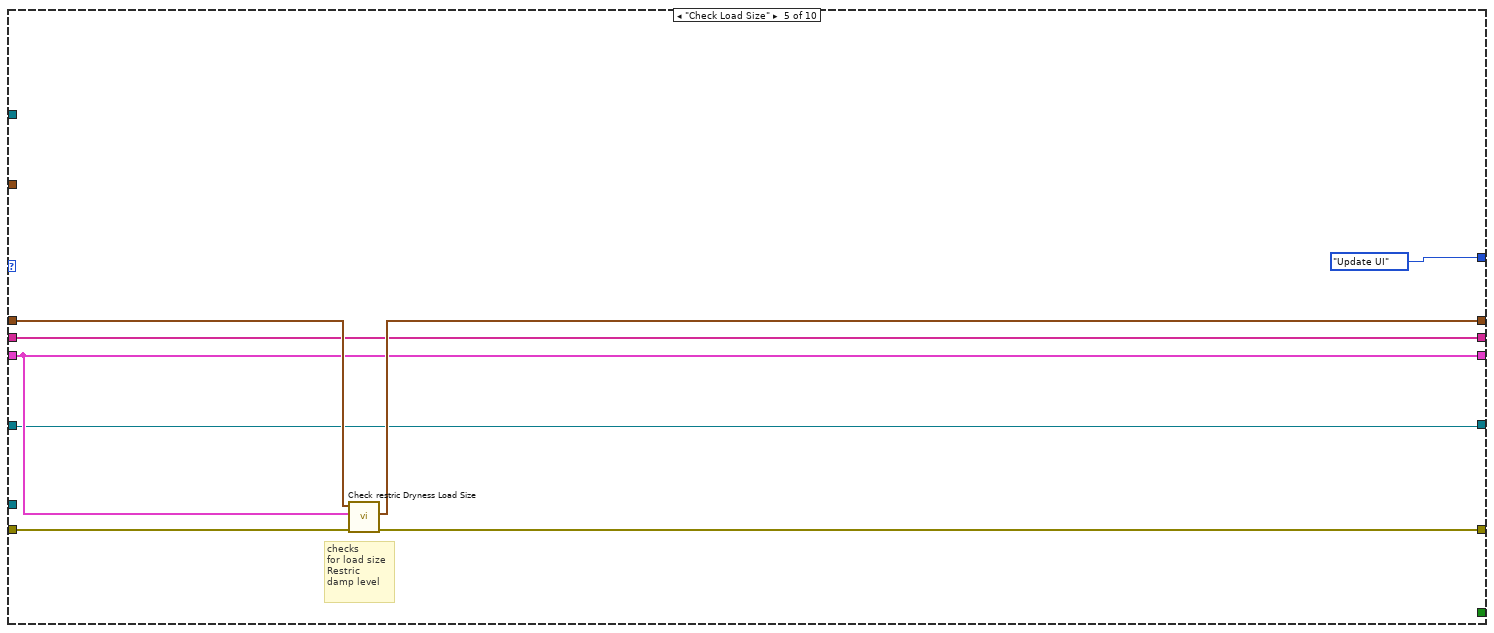
[diagram p9: hidden frame]
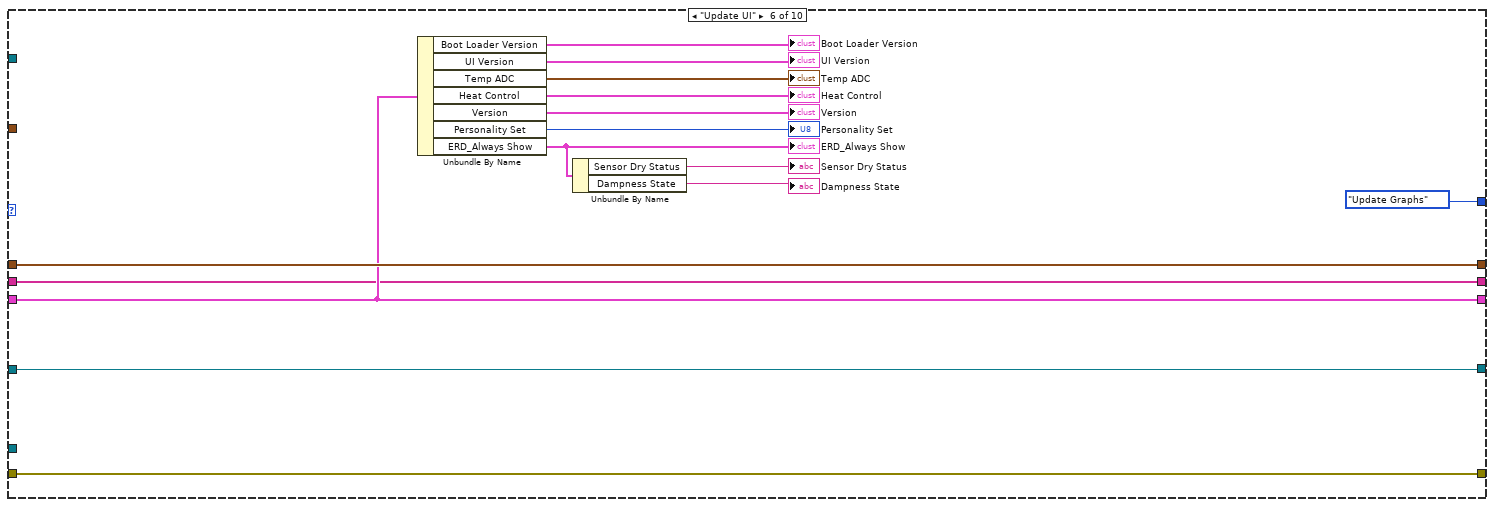
[diagram p10: hidden frame]
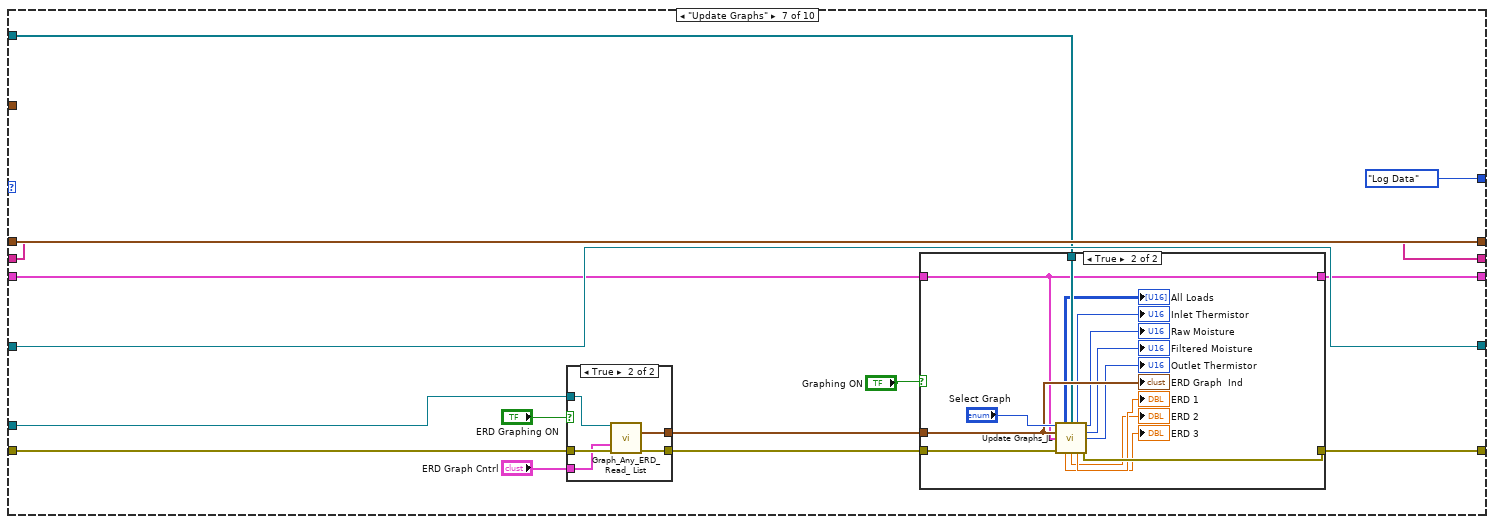
[diagram p11: hidden frame]
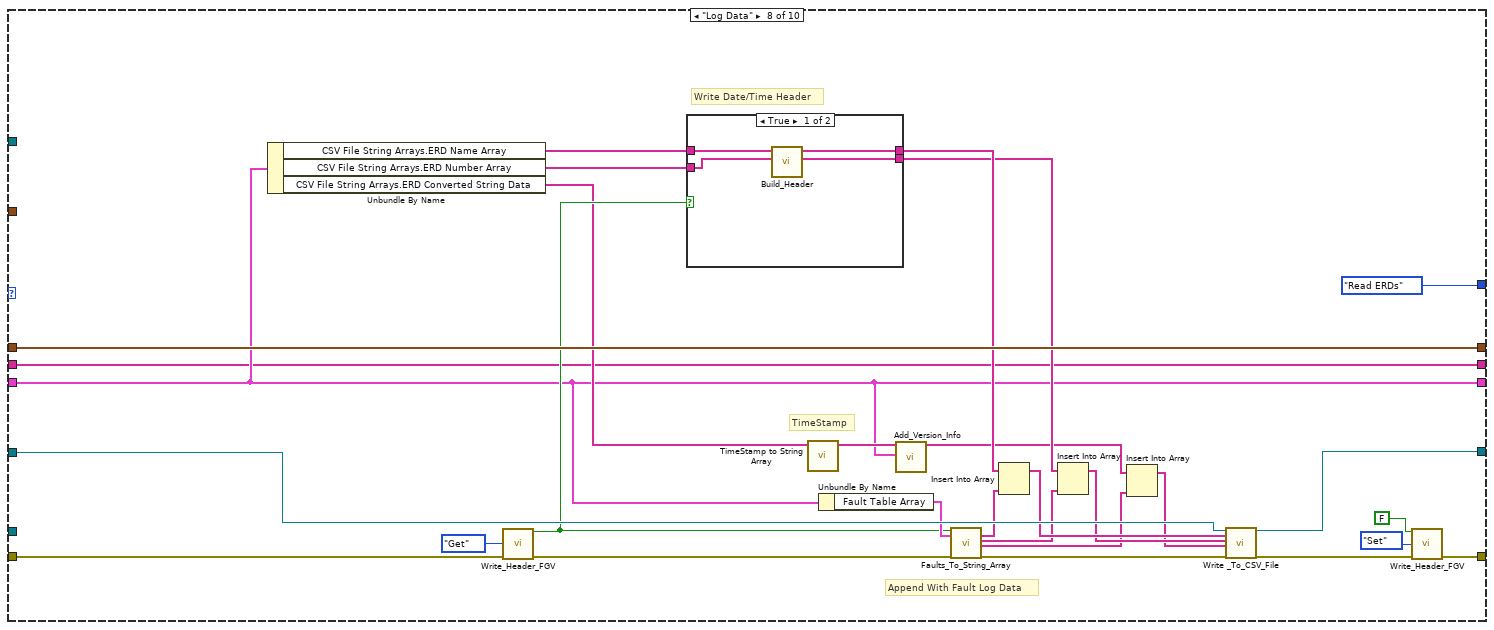
[diagram p14: hidden frame]
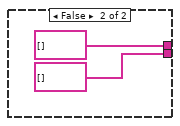
[diagram p15: hidden frame]
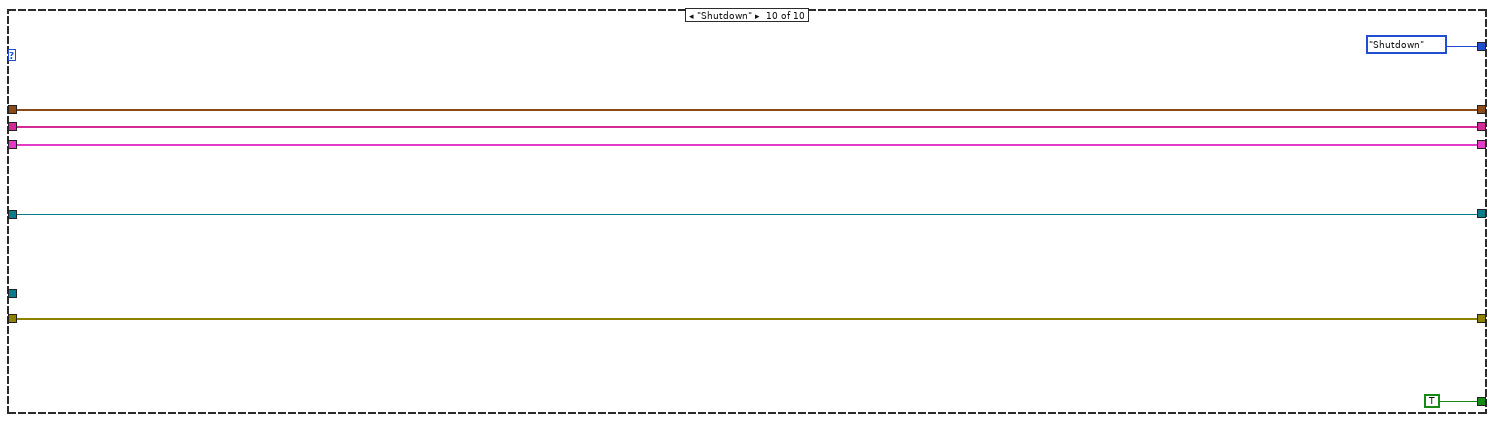
[diagram p16: hidden frame]
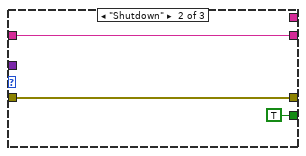
[diagram p18: hidden frame]
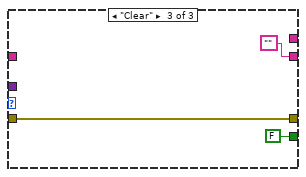
[diagram p19: hidden frame]
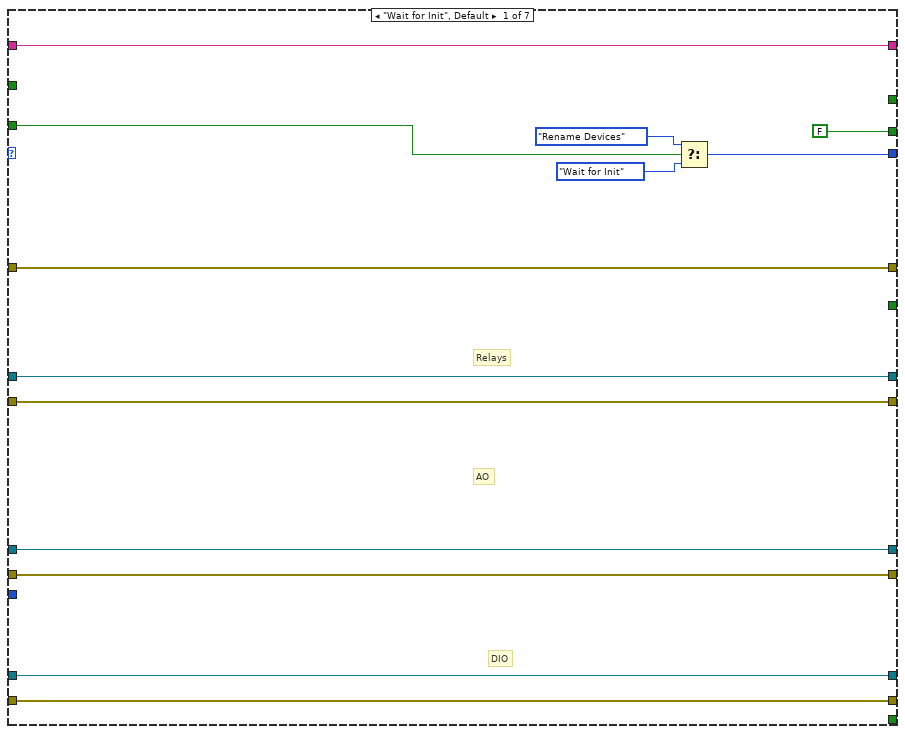
[diagram p20: hidden frame]
diagram:
  # "Get number of NewFIs connected\nand set this to the max value"
  n1 = Two Button Dialog(message="Are you using a Soft Load Box?" ("T button name (\"OK\")"), 1:"No" ("F button name (\"Cancel\")"), 2:"Yes" ("message")) -> (T button?=w17:bool)
  n2 = call "Is SLB FG.vi"("Error In"="Error In", "Action"=enum16{"Get", "Set"}."Set", "SLB?"=w17) -> ("Error Out"=w22:errorcluster, "SLB"=w21:bool)  [unwired: 7 in]
  n3 = case shown="True" w21 {
    tunnel: w22 -> [w32 w38]
    tunnel: [w32 w34] -> w14
    tunnel: path "C:/Automation/Configurations/JusticeLeague.ini" ("Config File Path") -> [_ w39]
    tunnel: "JL_SLB" ("cDAQ Name") -> [_ w36]
    tunnel: string[] ["9401_1", "9481_1", "9263_1"] ("Device List") -> [_ w35]
    frame False {
    }
    frame True {
      n4 = call "JLConfig Parse.vi"("Config File Path"=w39, "Error In"=w38) -> ("Calibrate"=w41:bool, "Error Out"=w40:errorcluster)  [unwired: 9 in, 3 out]
      n5 = property on="Scalling" class="Clust (strict)"(error in=w40, "Visible"=w41) -> (error out=w33:errorcluster)  [unwired: 1 in, 1 out]
      n6 = call "Rename DAQ Devices.vi"("cDAQ Name"=w36, "Error In"=w33) -> ("Error Out"=w37:errorcluster)  [unwired: 13 in]
      n7 = call "DeviceListCheck.vi"("Device List"=w35, "Error In"=w37) -> ("Error Out"=w34:errorcluster)  [unwired: 11 in, 2 out]
    }
  }
  n8 = call "Set Get Model.vi"("Error In"=w14, "Action"=enum16{"Set Model", "Get Model"}."Set Model", "Model"=enum16{"Estar Centauro", "GFL"}."Estar Centauro") -> ("Error Out"=w13:errorcluster)  [unwired: 7 in, 1 out]
  n9 = call "HEUI_Running_FGV.vi"("Running?"=FALSE, "Action"=enum16{"Get", "Set"}."Set", "Error In"=w13) -> ("Error Out"=w29:errorcluster)  [unwired: 11 in, 1 out]
  n10 = call "Get NEW FI Set Max.vi"("error in (no error)"=w29) -> ("Error Out"=w9:errorcluster, "Get Max_Out"=w10:dbl)  [unwired: 9 in]
  n11 = property on="Board Index" class="DigNum (strict)"(error in=w9, "Minimum"=w10) -> (error out=w7:errorcluster)  [unwired: 1 in, 1 out]
  n12 = call "GEA2 Initialize.vi"("Board Index"="Board Index", "Source Address"=u8 228, "error in"=w7) -> ("GEA2 Reference Out"=w5:refnum<k24>, "Board ID"=→"Board ID":string, "error out"=w2:errorcluster)  [unwired: 10 in]
  n13 = invoke class="GeaNode" method="RegisterAddress"(reference=w5, error in=w2, "address"=u8 229 ("Source Address")) -> (reference out=w3:refnum<k24>, error out=w4:errorcluster)  [unwired: 1 in, 2 out]
  n14 = case shown="No Error" w4 {
    selector: w4 -> [w109 w1405]
    tunnel: [w111 w1405] -> w31
    tunnel: w3 -> [w61 _]
    frame No Error {
      w44 = T47 {"Source"=0, "Destination"=0, "Command"=0, "Length"=0, "CRC"=0, "Message"=""}  # Data_Sent
      w43 = T47 {"Source"=0, "Destination"=0, "Command"=0, "Length"=0, "CRC"=0, "Message"=""}  # Data_Recv
      w52 = errorcluster {"status"=FALSE, "code"=0, "source"=""}  # Receive Loop Error
      w66 = refnum<k21> refnum ("task out")
      # "store user event in functional\nglobal variable, this will be used\nin the HEUI VI to obtain the proper\nuser event reference"
      # "Store initial GEA2 reference"
      n15 = call "FGV_GEA2_Ref.vi"("GEA2 Reference In"=w61, "Action"=enum16{"Set Ref", "Get Ref"}."Set Ref", "Error In"=w109) -> ("GEA2 Reference Out"=w55:refnum<k24>, "Error Out"=w42:errorcluster)  [unwired: 11 in]
      n16 = vi-ref "LabVIEW_GEA2_Toolkit.lvlibp:GEA2 Message Sent Event Handler.vi"() -> (w53:refnum<vi>)
      n17 = vi-ref "LabVIEW_GEA2_Toolkit.lvlibp:GEA2 Message Received Event Handler.vi"() -> (w54:refnum<vi>)
      n18 = Create User Event(user event datatype=w43, error in=w42) -> (user event=w48:refnum<user-event>, error out=w57:errorcluster)
      n19 = node(w57, w55, w54, w48) -> (w58:errorcluster)  [unwired: 1 in, 1 out]
      n20 = Create User Event(user event datatype=w44, error in=w58) -> (user event=w49:refnum<user-event>, error out=w56:errorcluster)
      n21 = node(w56, w55, w53, w49) -> (w51:errorcluster)  [unwired: 1 in, 1 out]
      n22 = Create User Event(user event datatype=w52, error in=w51) -> (user event=w45:refnum<user-event>, error out=w50:errorcluster)
      n23 = register-events(error in=w50, w48, w49, w45) -> (reference out=w47:refnum<event-registration>, error out=w46:errorcluster)  [unwired: 1 in]
      n24 = call "UI Loop Error and Que Setup.vi"("error in (no error)"=w46, "Receive Loop"=w45) -> ("error out"=w62:errorcluster, "UI Loop Event Registration"=w60:refnum<event-registration>, "Continuous Send Queue"=w82:refnum<queue>, "GEA Display Queue"=w63:refnum<queue>, "Daq Loop queue"=w65:refnum<queue>, "ERD Queue Loop"=w64:refnum<queue>)  [unwired: 4 in]
      n25 = call "Get User Filename and Path.vi"("error in (no error)"=w62) -> ("error out"=w72:errorcluster, "TXT File Path"=w78:path, "CSV File Path"=w80:path)  [unwired: 8 in]
      n26 = control-ref of="All Loads"() -> (w67:refnum<vi>)
      n27 = control-ref of="Inlet Thermistor"() -> (w68:refnum<vi>)
      n28 = control-ref of="Outlet Thermistor"() -> (w69:refnum<vi>)
      n29 = control-ref of="Raw Moisture"() -> (w70:refnum<vi>)
      n30 = control-ref of="Filtered Moisture"() -> (w71:refnum<vi>)
      n31 = control-ref of="ERD 1"() -> (w97:refnum<vi>)
      n32 = control-ref of="ERD 2"() -> (w95:refnum<vi>)
      n33 = control-ref of="ERD 3"() -> (w96:refnum<vi>)
      n34 = Create User Event(user event datatype=TRUE ("Bool"), error in=w62) -> (user event=w104:refnum<user-event>, error out=w105:errorcluster)
      n35 = call "Open_Create__Log_File.vi"("File Path Control"=w80, "Enum"=enum16{"CSV File", "Text File"}."CSV File", "Error In"=w72) -> ("refnum out"=w98:refnum<file>, "File Path"=→"CSV File Log Path":path, "Error Out"=w107:errorcluster)  [unwired: 10 in]
      n36 = call "Open_Create__Log_File.vi"("File Path Control"=w78, "Enum"=enum16{"CSV File", "Text File"}."Text File", "Error In"=w72) -> ("refnum out"=w77:refnum<file>, "Error Out"=w79:errorcluster)  [unwired: 10 in, 1 out]
      n37 = call "HEUI_Event_FGV.vi"("Event In"=w104, "Action"=enum16{"Get", "Set"}."Set", "Error In"=w105) -> ("Event Out"=w101:refnum<user-event>, "Error Out"=w102:errorcluster)  [unwired: 11 in]
      n38 = Unbundle By Name(T37 {"Data"=variant, "State"=enum."Init"} ("Data")) -> ("State"=w99:T38)
      n39 = Build Array(w67, w68, w69, w70, w71, w97, w95, w96) -> (w94:refnum<vi>[])
      n40 = while "Periodic ERD Query Loop" {
        shift-right: [w190] -> w91
        shift-left: w107 -> [w192]
        tunnel: w64 -> [w193]
        shift-right: [w184] -> _
        shift-left: w99 -> [w186]
        shift-right: [w179] -> _
        shift-left: _ -> [w178]
        tunnel: w98 -> [w177]
        tunnel: [w176] -> w89
        shift-right: [w175] -> _
        shift-left: _ -> [w174]
        tunnel: w94 -> [w173]
        shift-right: [w171] -> _
        shift-left: _ -> [w170]
        stop <- w189 stop-if-true
        # "ERD Loop"
        n41 = Dequeue Element(queue=w193, timeout in ms (-1)=0, error in (no error)=w192) -> (element=w181:T37, timed out?=w172:bool, error out=w191:errorcluster)  [unwired: 1 out]
        n42 = Unbundle By Name(w181) -> ("State"=w187:T38)
        n43 = call "FGV_GEA2_Ref.vi"("Action"=enum16{"Set Ref", "Get Ref"}."Get Ref", "Error In"=w191) -> ("GEA2 Reference Out"=w180:refnum<k24>, "Error Out"=w183:errorcluster)  [unwired: 12 in]
        n44 = Select(t=w186, s=w172, f=w187) -> (s? t:f=w185:T38)
        n45 = case shown="\"Pause\"" w185 {
          tunnel: w183 -> [w203 w211 w218 w246 w262 w272 w289 w337 w355 w362]
          tunnel: [w196 w208 w227 w241 w260 w272 w287 w334 w355 w362] -> w188
          tunnel: [_ _ _ _ _ _ _ _ _ TRUE] -> w189
          tunnel: "ERD Spam GEA Inputs" -> [_ _ w223 _ _ _ _ _ _ _]
          tunnel: [ERD_Loop_States_JL."Build ERD Read List" ("State") ERD_Loop_States_JL."Read ERDs" ("State") ERD_Loop_States_JL."Get Version" ("State") ERD_Loop_States_JL."Check Load Size" ("State") ERD_Loop_States_JL."Update UI" ("State") ERD_Loop_States_JL."Update Graphs" ("State") ERD_Loop_States_JL."Log Data" ("State") ERD_Loop_States_JL."Read ERDs" ("t") ERD_Loop_States_JL."Pause" ("State") ERD_Loop_States_JL."Shutdown" ("State")] -> w184
          tunnel: w180 -> [_ _ w222 w251 _ _ w282 _ _ _]
          tunnel: [w201 w210 w215 w253 w259 w276 w291 w343 w353 w359] -> w179
          tunnel: w178 -> [w201 _ w215 w253 w261 w276 w291 w343 w353 w359]
          tunnel: w177 -> [w200 w207 w231 w252 w257 w273 w290 w342 w352 w358]
          tunnel: [w200 w207 w231 w252 w257 w273 w290 w341 w352 w358] -> w176
          tunnel: [w199 w206 w226 w242 w258 w274 w280 w316 w351 w357] -> w175
          tunnel: w174 -> [w199 w206 _ w248 w258 w274 w281 w316 w351 w357]
          tunnel: w173 -> [_ _ _ _ _ _ w283 _ _ _]
          tunnel: [w195 w205 w216 w238 w255 w263 w278 w315 w350 w356] -> w171
          tunnel: w170 -> [w195 _ w216 w238 w255 w263 w278 w315 w350 w356]
          frame "Init", Default {
            # "Set Write Header\nFGV to True"
            n46 = call "Write_Header_FGV.vi"("Write Header ? In"=TRUE, "Action"=enum16{"Get", "Set"}."Set", "Error In"=w203) -> ("Error Out"=w196:errorcluster)  [unwired: 11 in, 1 out]
          }
          frame "Build ERD Read List" {
            n47 = call "ERD_Read_List_Builder.vi"("ERD Read List"="ERD Read List", "Error In"=w211) -> ("Read ERD List"=w210:T12[], "ERD Name"=w205:string[], "Error Out"=w208:errorcluster)  [unwired: 15 in]
          }
          frame "Read ERDs" {
            n48 = local read "Model"() -> (w221:enum16{"Estar Centauro", "GFL"})
            n49 = Equal?(x=w221, y=enum16{"Estar Centauro", "GFL"}."GFL") -> (x = y?=w214:bool)
            n50 = Select(t=1 ("#ERDs per message"), s=w214, f=2) -> (s? t:f=w217:i32)
            n51 = call "Add Version Data to  ERD list.vi"(".NET Refnum in"=w222, "# of Iterations (Should be 2 except JL)"=w217, "GEA Inputs"=w223, "Read ERD List MC"=w215, "error in (no error)"=w218, "#ERDs per message"="#ERDs per message") -> ("ERD Data Out out"=w225:T48[], "error out"=w224:errorcluster)  [unwired: 8 in]
            n52 = call "Write_Header_FGV.vi"("Action"=enum16{"Get", "Set"}."Get", "Error In"=w224) -> ("Write Header ? Out"=w228:bool, "Error Out"=w230:errorcluster)  [unwired: 12 in]
            n53 = call "Convert_ERDs_JL.vi"("New Header?"=w228, "ERD Name"=w216, "Array"=w225, "Error In"=w230) -> ("All_ERD_Data_Bundled_Brass"=w226:T49, "Error Out"=w227:errorcluster)  [unwired: 10 in]
          }
          frame "Get Version" {
            n54 = call "GEA2 Send and Receive Message.vi"("GEA2 Reference In"=w251, "Input Data"=T9 {"Source"=229, "Destination"=36, "Command"=1, "Message"=""}, "Expected Command"="01", "Expected Source"="24", "Error In"=w246) -> ("GEA2 Reference Out"=w245:refnum<k24>, "Converted Data Out"=w249:T47, "Error Out"=w247:errorcluster)  [unwired: 7 in, 1 out]
            n55 = call "Version_Parse.vi"("All_ERD_Data_Bundled_Brass in"=w248, "Converted Data Out"=w249, "Error In"=w247) -> ("All_ERD_Data_Bundled_Brass out"=w244:T49, "Error Out"=w243:errorcluster)  [unwired: 11 in]
            n56 = call "GEA2 Send and Receive Message.vi"("GEA2 Reference In"=w245, "Input Data"=T9 {"Source"=229, "Destination"=37, "Command"=1, "Message"=""}, "Expected Command"="01", "Expected Source"="25", "Error In"=w243) -> ("Converted Data Out"=w235:T47, "Error Out"=w236:errorcluster)  [unwired: 7 in, 2 out]
            n57 = call "Version_Parse.vi"("All_ERD_Data_Bundled_Brass in"=w244, "Converted Data Out"=w235, "Error In"=w236) -> ("All_ERD_Data_Bundled_Brass out"=w242:T49, "Error Out"=w241:errorcluster)  [unwired: 11 in]
          }
          frame "Check Load Size" {
            # "checks \nfor load size \nRestric\ndamp level"
            n58 = call "Check restric Dryness Load Size.vi"("Error In"=w262, "All_ERD_Data_Bundled_Brass out"=w258, "Read ERD List"=w261) -> ("Error Out"=w260:errorcluster, "New ERD Data"=w259:T12[])  [unwired: 7 in]
          }
          frame "Update UI" {
            n59 = Unbundle By Name(w274) -> ("Boot Loader Version"=→"Boot Loader Version":T4, "UI Version"=→"UI Version":T5, "Temp ADC"=→"Temp ADC":T1, "Heat Control"=→"Heat Control":T28, "Version"=→"Version":T50, "Personality Set"=→"Personality Set":u8, "ERD_Always Show"=w271:T2)
            "ERD_Always Show" <- w271
            n60 = Unbundle By Name(w271) -> ("Sensor Dry Status"=→"Sensor Dry Status":string, "Dampness State"=→"Dampness State":string)
          }
          frame "Update Graphs" {
            n61 = case shown="True" "ERD Graphing ON" {
              tunnel: w289 -> [w309 w314]
              tunnel: [w309 w313] -> w288
              tunnel: "ERD Graph Cntrl" -> [_ w312]
              tunnel: [_ w311] -> w284
              tunnel: w282 -> [_ w310]
              frame False {
              }
              frame True {
                n62 = call "Graph_Any_ERD_ Read_ List.vi"("GEA2 Reference In"=w310, "ERD Graph Cntrl"=w312, "Error In"=w314) -> ("ERD Graph  Ind"=w311:T15, "Error Out"=w313:errorcluster)  [unwired: 10 in, 1 out]
              }
            }
            n63 = case shown="True" "Graphing ON" {
              tunnel: w288 -> [w293 w308]
              tunnel: [w293 w307] -> w287
              tunnel: w284 -> [_ w305]
              tunnel: w283 -> [_ w304]
              tunnel: w281 -> [w294 w300]
              tunnel: [w294 w300] -> w280
              frame False {
              }
              frame True {
                n64 = call "Update Graphs_JL.vi"("Select Graph"="Select Graph", "appended array"=w304, "ERD Graph  Ind 2"=w305, "ERD_Data_Bundled_In"=w300, "Error In"=w308) -> ("All Loads"=→"All Loads":u16[][], "Inlet Thermistor"=→"Inlet Thermistor":u16, "Raw Moisture"=→"Raw Moisture":u16, "Filtered Moisture"=→"Filtered Moisture":u16, "Outlet Thermistor"=→"Outlet Thermistor":u16, "ERD 3"=→"ERD 3":dbl, "ERD 2"=→"ERD 2":dbl, "ERD 1"=→"ERD 1":dbl, "Error Out"=w307:errorcluster)  [unwired: 2 in]
                "ERD Graph  Ind" <- w305
              }
            }
          }
          frame "Log Data" {
            # "TimeStamp"
            # "Append With Fault Log Data"
            # "Write Date/Time Header"
            n65 = Unbundle By Name(w316) -> ("CSV File String Arrays.ERD Name Array"=w340:string[], "CSV File String Arrays.ERD Number Array"=w339:string[], "CSV File String Arrays.ERD Converted String Data"=w318:string[])
            n66 = call "Write_Header_FGV.vi"("Action"=enum16{"Get", "Set"}."Get", "Error In"=w337) -> ("Write Header ? Out"=w319:bool, "Error Out"=w332:errorcluster)  [unwired: 12 in]
            n67 = case shown="True" w319 {
              tunnel: w340 -> [w344 _]
              tunnel: [w346 string[] [] ("ERD Name Array")] -> w331
              tunnel: w339 -> [w345 _]
              tunnel: [w347 string[] [] ("ERD Number Array")] -> w329
              frame True {
                n68 = call "Build_Header.vi"("ERD Number Array In"=w345, "ERD Name Array In"=w344) -> ("ERD Number Array out"=w347:string[], "ERD Name Array out"=w346:string[])  [unwired: 8 in]
              }
              frame False {
              }
            }
            n69 = call "TimeStamp to String Array.vi"("String Array In"=w318) -> ("String Array Out"=w317:string[])  [unwired: 10 in]
            n70 = Unbundle By Name(w316) -> ("Fault Table Array"=w321:T52)
            n71 = call "Add_Version_Info.vi"("String Array In"=w317, "All_ERD_Data_Bundled_Brass out"=w316) -> ("String Array Out"=w327:string[])  [unwired: 17 in]
            n72 = call "Faults_To_String_Array.vi"("Write Header ?"=w319, "Fault Table Entry"=w321, "Error In"=w332) -> ("Fault Header String Array"=w326:string[], "Fault ERD Number String Array"=w325:string[], "Fault Data String Array"=w324:string[], "Error Out"=w322:errorcluster)  [unwired: 13 in]
            n73 = Insert Into Array(array=w331, new element=w326) -> (w330:string[])  [unwired: 1 in]
            n74 = Insert Into Array(array=w329, new element=w325) -> (w328:string[])  [unwired: 1 in]
            n75 = Insert Into Array(array=w327, new element=w324) -> (w323:string[])  [unwired: 1 in]
            n76 = call "Write _To_CSV_File.vi"("Refnum In"=w342, "String Array 1"=w330, "String Array 2"=w328, "String Array 3"=w323, "Error In"=w322) -> ("Refnum Out"=w341:refnum<file>, "Error Out"=w335:errorcluster)  [unwired: 12 in, 1 out]
            n77 = call "Write_Header_FGV.vi"("Write Header ? In"=FALSE, "Action"=enum16{"Get", "Set"}."Set", "Error In"=w335) -> ("Error Out"=w334:errorcluster)  [unwired: 11 in, 1 out]
          }
          frame "Pause" {
          }
          frame "Shutdown" {
          }
        }
        n78 = Tick Count (ms)() -> ()  [unwired: 1 out]
        n79 = call "Error_Control.vi"("Error In"=w188) -> ("Error Out"=w190:errorcluster)  [unwired: 14 in]
      }
      n80 = while "UI Loop" {
        shift-right: [w656] -> w134
        shift-left: w102 -> [w650]
        shift-right: [w658] -> w133
        shift-left: _ -> [_]
        tunnel: w60 -> [w657]
        tunnel: w101 -> [w647]
        tunnel: w64 -> [w646]
        tunnel: w47 -> [w645]
        stop <- w655 stop-if-true
        # "UI Loop"
        n81 = call "FGV_GEA2_Ref.vi"("Action"=enum16{"Set Ref", "Get Ref"}."Get Ref", "Error In"=w650) -> ("GEA2 Reference Out"=w649:refnum<k24>, "Error Out"=w651:errorcluster)  [unwired: 12 in]
        n82 = event shown="[6] \"Read ERD\": Value Change" {
          selector: w657 -> [_ _ _ _ _ _ _ _ _ _ _ _ _ _ _ _ _ _ _ _ _ _ _ _ _ _ _ _ _ _]
          dyn-events: _ -> [_ _ _ _ _ _ _ _ _ _ _ _ _ _ _ _ _ _ _ _ _ _ _ _ _ _ _ _ _ _]
          timeout: 100 -> [_ _ _ _ _ _ _ _ _ _ _ _ _ _ _ _ _ _ _ _ _ _ _ _ _ _ _ _ _ _]
          tunnel: [w662 w670 w676 w688 w695 w709 w712 w727 w740 w753 w796 w849 w855 w870 w921 w962 w966 w976 _ w991 w1035 w1125 w1206 w1208 w1228 w1259 w1272 w1302 w1312 w1325] -> w654
          tunnel: w651 -> [w659 w667 w674 w688 w690 w704 w711 w726 w747 w761 w801 w854 w865 w872 w923 w964 w970 w977 w982 w988 w1037 w1127 w1204 w1211 w1229 w1258 w1269 w1303 w1320 w1325]
          tunnel: [_ _ _ _ _ _ _ _ _ _ _ _ _ _ _ _ _ _ _ _ _ _ _ _ _ _ _ _ TRUE _] -> w655
          tunnel: w649 -> [w660 w669 w680 w689 w693 w706 w715 _ w746 w762 w802 w853 w864 w868 w920 w957 _ w975 _ w1000 w1038 w1128 _ w1210 w1226 w1261 w1270 _ w1323 w1326]
          tunnel: [w663 w669 _ w689 w696 w710 w716 _ w745 _ _ _ w863 w867 w919 w956 _ w975 _ _ w1034 w1124 _ w1209 w1227 w1260 w1271 _ w1323 w1326] -> w658
          tunnel: "GEA Inputs" -> [_ _ w679 _ w694 w705 w714 _ w744 _ _ _ _ w866 w918 w959 _ _ _ _ w1039 w1129 _ w1212 w1230 w1262 w1273 _ _ _]
          tunnel: w647 -> [_ _ _ _ _ _ _ _ _ w758 w800 _ _ _ _ _ _ _ _ w985 _ _ _ _ _ _ _ _ _ _]
          tunnel: w646 -> [_ _ w675 _ _ _ _ _ _ w752 w797 w848 _ _ _ w961 _ _ _ w986 _ _ w1202 _ _ _ _ w1300 _ _]
          tunnel: w645 -> [_ _ _ _ _ _ _ _ _ _ _ _ _ _ _ _ _ _ _ _ _ _ _ _ _ _ _ _ _ _]
          event "Send Button": Value Change {
            n83 = event-data() -> ()  [unwired: 1 in, 1 out]
            n84 = call "GEA2 Send Message.vi"("GEA2 Reference In"=w660, "Input Data"="GEA2 Send", "Error In"=w659) -> ("GEA2 Reference Out"=w663:refnum<k24>, "Error Out"=w662:errorcluster)  [unwired: 11 in]
          }
          event "Clear": Value Change {
            w664 = T40 {"Data"=variant, "State"=enum."Clear"} ("element")
            n85 = event-data() -> ()  [unwired: 1 in, 6 out]
            n86 = Obtain Queue(name (unnamed)="GEA2", element data type=w664, error in (no error)=w667) -> (queue out=w665:refnum<queue>, error out=w668:errorcluster)  [unwired: 2 in, 1 out]
            n87 = Enqueue Element(queue=w665, element=w664, error in (no error)=w668) -> (error out=w670:errorcluster)  [unwired: 1 in, 2 out]
          }
          event "Set Personality": Value Change {
            n88 = event-data() -> ()  [unwired: 1 in, 6 out]
            n89 = Index Array(array=T42[] [{"ERD Number"=61733, "Data Type"=enum."string", "Data"=""}] ("Write ERD List")) -> (element=w685:T42)  [unwired: 1 in]
            n90 = Number To Hexadecimal String(1:i16 2 ("width (-)"), 2:"?") -> (0:w684:string)
            n91 = Bundle By Name(cluster=w685, "Data"=w684) -> (w683:T42)
            n92 = Build Array(w683) -> (w682:T42[])
            n93 = call "GEA2 Write ERD.vi"("GEA2 Reference In"=w680, "GEA Inputs"=w679, "Write ERD List"=w682, "Error In"=w674, "Verify ERD Response?"=TRUE) -> ("Error Out"=w672:errorcluster)  [unwired: 8 in, 2 out]
            n94 = control-ref of="Board Index 2"() -> ()  [unwired: 1 out]
            n95 = call "Get NEW FI Set Max.vi"("error in (no error)"=w672) -> ("Error Out"=w671:errorcluster)  [unwired: 9 in, 1 out]
            n96 = call "FGV_GEA2_Ref.vi"("Action"=enum16{"Set Ref", "Get Ref"}."Get Ref", "Error In"=w671) -> ()  [unwired: 12 in, 2 out]
            n97 = Enqueue Element(queue=w675, element=T37 {"Data"=variant, "State"=enum."Init"} ("Data")) -> (error out=w676:errorcluster)  [unwired: 2 in, 2 out]
          }
          event Timeout {
            # "Must have timeout case to give GEA2 FGV a chance to update\nthe GEA2 reference. Otherwise, when we receive an event it may\nbe using a reference that is no longer valid."
            n98 = event-data() -> ()  [unwired: 1 in, 3 out]
          }
          event "Write ERD": Value Change {
            n99 = event-data() -> ()  [unwired: 1 in, 1 out]
            n100 = call "GEA2 Write ERD.vi"("GEA2 Reference In"=w693, "# of Tries"=2 ("Retry Count"), "GEA Inputs"=w694, "Write ERD List"="Write ERD List", "Error In"=w690, "Verify ERD Response?"=TRUE) -> ("GEA2 Reference Out"=w696:refnum<k24>, "Error Out"=w695:errorcluster)  [unwired: 7 in, 1 out]
          }
          event "Enable CC Mode": Value Change {
            n101 = event-data() -> ()  [unwired: 1 in, 1 out]
            n102 = call "JL_Continuous Cycle Mode Config.vi"("GEA2 Reference In"=w706, "Completed Cycles"="Completed Cycles", "Enabled"="Enabled", "GEA Inputs"=w705, "TimeBetween Cycles"="TimeBetween Cycles", "Requested Cycles"="Requested Cycles", "Error In"=w704) -> ("GEA2 Reference Out"=w699:refnum<k24>, "Error Out"=w698:errorcluster)  [unwired: 6 in, 1 out]
            n103 = call "GEA2 Write ERD.vi"("GEA2 Reference In"=w699, "# of Tries"=2 ("Retry Count"), "GEA Inputs"=w705, "Write ERD List"=T42[] [{"ERD Number"=61770, "Data Type"=enum."string", "Data"="01"}], "Error In"=w698) -> ("GEA2 Reference Out"=w710:refnum<k24>, "Error Out"=w709:errorcluster)  [unwired: 8 in, 1 out]
          }
          event "Read ERD": Value Change {
            n104 = event-data() -> ()  [unwired: 1 in, 6 out]
            n105 = call "GEA2 Read ERD.vi"("GEA2 Reference In"=w715, "Retry Count"=2, "GEA Inputs"=w714, "Read ERD List"="Read ERD List", "Error In"=w711, "Verify ERD Response?"=TRUE) -> ("GEA2 Reference Out"=w716:refnum<k24>, "ERD Data Out"=→"Read ERD Data Out":T48[], "Error Out"=w712:errorcluster)  [unwired: 6 in, 1 out]
          }
          event "UI Launch": Value Change {
            n106 = event-data() -> ()  [unwired: 1 in, 6 out]
            n107 = call "HEUI_Running_FGV.vi"("Action"=enum16{"Get", "Set"}."Get", "Error In"=w726) -> ("Running?"=w723:bool, "Error Out"=w725:errorcluster)  [unwired: 12 in]
            n108 = Current VI's Path() -> (path=w721:path)
            n109 = Strip Path(path=w721) -> (stripped path=w722:path)  [unwired: 1 out]
            n110 = case shown="False" w723 {
              tunnel: w725 -> [w737 w739]
              tunnel: [w736 w739] -> w727
              tunnel: w722 -> [w729 _]
              tunnel: "UI Launch" -> [_ _]
              frame False {
                w738 = 128  # options
                n111 = Build Path(base path=w729, name or relative path="JLMainUI.vi") -> (appended path=w734:path)
                n112 = Open VI Reference(type specifier VI Refnum (for type only)=refnum<vi> refnum, vi path=w734, options=w738, error in (no error)=w737) -> (vi reference=w731:refnum<vi>, error out=w733:errorcluster)  [unwired: 2 in]
                n113 = call-by-ref "Start Asynchronous Call"(reference=w731, error in=w733) -> (reference out=w730:refnum<vi>, error out=w732:errorcluster)  [unwired: 10 in, 2 out]
                n114 = Close Reference(reference=w730, error in (no error)=w732) -> (error out=w736:errorcluster)
              }
              frame True {
              }
            }
          }
          event "Read Parametric": Value Change {
            n115 = event-data() -> ()  [unwired: 1 in, 6 out]
            n116 = call "Para_ERD_Fxxx.vi"("GEA Inputs"=w744, "Error In"=w747, "Read ERD List"=T12[] [{"ERD Number"=62976, "Data Type"=enum."string"}, {"ERD Number"=62977, "Data Type"=enum."string"}, {"ERD Number"=63015, "Data Type"=enum."string"}, {"ERD Number"=63016, "Data Type"=enum."string"}, {"ERD Number"=63017, "Data Type"=enum."string"}, {"ERD Number"=63018, "Data Type"=enum."string"}, {"ERD Number"=63019, "Data Type"=enum."string"}, {"ERD Number"=63020, "Data Type"=enum."string"}, {"ERD Number"=63021, "Data Type"=enum."string"}, {"ERD Number"=63022, "Data Type"=enum."string"}, {"ERD Number"=63023, "Data Type"=enum."string"}, {"ERD Number"=63024, "Data Type"=enum."string"}, {"ERD Number"=63025, "Data Type"=enum."string"}, {"ERD Number"=63026, "Data Type"=enum."string"}, {"ERD Number"=63028, "Data Type"=enum."string"}, {"ERD Number"=63029, "Data Type"=enum."string"}, {"ERD Number"=63030, "Data Type"=enum."string"}, {"ERD Number"=63031, "Data Type"=enum."string"}, {"ERD Number"=63032, "Data Type"=enum."string"}, {"ERD Number"=63033, "Data Type"=enum."string"}, {"ERD Number"=63034, "Data Type"=enum."string"}, {"ERD Number"=63035, "Data Type"=enum."string"}, {"ERD Number"=63036, "Data Type"=enum."string"}, {"ERD Number"=63037, "Data Type"=enum."string"}, {"ERD Number"=63038, "Data Type"=enum."string"}, {"ERD Number"=63039, "Data Type"=enum."string"}, {"ERD Number"=63040, "Data Type"=enum."string"}, {"ERD Number"=63041, "Data Type"=enum."string"}, {"ERD Number"=63042, "Data Type"=enum."string"}, {"ERD Number"=63043, "Data Type"=enum."string"}, {"ERD Number"=63044, "Data Type"=enum."string"}, {"ERD Number"=63045, "Data Type"=enum."string"}, {"ERD Number"=63046, "Data Type"=enum."string"}, {"ERD Number"=63047, "Data Type"=enum."string"}, {"ERD Number"=63048, "Data Type"=enum."string"}, {"ERD Number"=63049, "Data Type"=enum."string"}, {"ERD Number"=63050, "Data Type"=enum."string"}, {"ERD Number"=63052, "Data Type"=enum."string"}, {"ERD Number"=63053, "Data Type"=enum."string"}, {"ERD Number"=63054, "Data Type"=enum."string"}, {"ERD Number"=63055, "Data Type"=enum."string"}, {"ERD Number"=63056, "Data Type"=enum."string"}, {"ERD Number"=63060, "Data Type"=enum."string"}, {"ERD Number"=63061, "Data Type"=enum."string"}, {"ERD Number"=63067, "Data Type"=enum."string"}, {"ERD Number"=63068, "Data Type"=enum."string"}, {"ERD Number"=63072, "Data Type"=enum."string"}, {"ERD Number"=63073, "Data Type"=enum."string"}, {"ERD Number"=63074, "Data Type"=enum."string"}, {"ERD Number"=63075, "Data Type"=enum."string"}, {"ERD Number"=63076, "Data Type"=enum."string"}, {"ERD Number"=63077, "Data Type"=enum."string"}, {"ERD Number"=63078, "Data Type"=enum."string"}, {"ERD Number"=63079, "Data Type"=enum."string"}, {"ERD Number"=63080, "Data Type"=enum."string"}, {"ERD Number"=63081, "Data Type"=enum."string"}], "GEA2 Reference In"=w746) -> ("Error Out"=w741:errorcluster, "F6XX"=w742:T54, "GEA2 Reference Out"=w745:refnum<k24>)  [unwired: 4 in, 1 out]
            n117 = call "Parametric Viewer.vi"("Error In"=w741, "F6XX_In"=w742) -> ("Error Out"=w740:errorcluster)  [unwired: 8 in, 1 out]
          }
          event Value Change {
            (unwired) "ERD Loop" ("name (unnamed)")
            w754 = TRUE ("Blinking")
            n118 = event-data() -> ()  [unwired: 1 in, 6 out]
            n119 = Generate User Event(user event=w758, event data cluster=TRUE ("event data"), error in=w761) -> (error out=w759:errorcluster)  [unwired: 1 in, 1 out]
            n120 = property on="Program Ind" class="Bool (strict)"(error in=w759, "Value"=w754, "Blinking"=w754) -> (error out=w755:errorcluster)  [unwired: 1 in, 1 out]
            n121 = Enqueue Element(queue=w752, element=T37 {"Data"=variant, "State"=enum."Pause"} ("Data"), error in (no error)=w755) -> (error out=w757:errorcluster)  [unwired: 1 in, 2 out]
            n122 = property on="GEA2 Send" class="Clust (strict)"() -> ("Value"=w750:T9)  [unwired: 2 in, 2 out]
            n123 = Unbundle By Name("Programming") -> ("File Path"=w765:path)
            n124 = call "Time Delay3"("error in (no error)"=w757, "Delay Time (s)"=2.0) -> ("error out"=w756:errorcluster)  [unwired: 9 in]
            n125 = Unbundle By Name(w750) -> ("Source"=w749:u8, "Destination"=w748:u8)
            n126 = Not Equal?(x=w765, y=path "") -> (x != y?=w764:bool)
            n127 = case shown="True" w764 {
              tunnel: w756 -> [w768 w773]
              tunnel: [w768 w780] -> w753
              tunnel: w765 -> [_ w785]
              tunnel: w762 -> [_ w781]
              tunnel: w749 -> [_ w770]
              tunnel: w748 -> [_ w769]
              frame False {
              }
              frame True {
                w771 = T8 9 items=["ImageRejected", "BoardNotFound", "UnableToGetGeaConfiguration", "WriteToFlashNotAllowed", "ImageDownloadedSuccessfully", "ImagePresent", "WriteToFlashFailed", "EraseFailed", "CrcFailed", ""] ("Result")
                w779 = FALSE ("Blinking")
                n128 = property on="Result" class="Ring (strict)"(error in=w773, "Value"=w771) -> (error out=w772:errorcluster)  [unwired: 1 in, 1 out]
                n129 = property on="Board Index" class="DigNum (strict)"(error in=w773, "DisabledEnum"=T41."Disabled and Grayed Out" ("Disabled")) -> ()  [unwired: 1 in, 2 out]
                n130 = call "GEA2 Flash APL.vi"("GEA2 Reference In"=w781, "Force Update?"=TRUE, "Source Address"=w770, "Destination Address"=w769, "File Path"=w785, "Error In"=w772, "Broadcast"=TRUE, "Reset?"=FALSE ("Reset Board?")) -> ("Result"=w774:i32, "Error Out"=w776:errorcluster)  [unwired: 3 in, 3 out]
                n131 = property on="Result" class="Ring (strict)"(error in=w776, "Value"=w774) -> (error out=w775:errorcluster)  [unwired: 1 in, 1 out]
                n132 = property on="Board Index" class="DigNum (strict)"(error in=w776, "DisabledEnum"=T41."Enabled" ("Disabled")) -> ()  [unwired: 1 in, 2 out]
                n133 = property on="Program Ind" class="Bool (strict)"(error in=w775, "Value"=w779, "Blinking"=w779) -> (error out=w780:errorcluster)  [unwired: 1 in, 1 out]
              }
            }
          }
          event "Flash Latest": Value Change {
            (unwired) "ERD Loop" ("name (unnamed)")
            w791 = TRUE ("Blinking")
            (unwired) FALSE ("Data On")
            n134 = event-data() -> ()  [unwired: 1 in, 6 out]
            n135 = Generate User Event(user event=w800, event data cluster=TRUE ("event data"), error in=w801) -> (error out=w793:errorcluster)  [unwired: 1 in, 1 out]
            n136 = property on="Program Ind" class="Bool (strict)"(error in=w793, "Value"=w791, "Blinking"=w791) -> (error out=w792:errorcluster)  [unwired: 1 in, 1 out]
            n137 = Enqueue Element(queue=w797, element=T37 {"Data"=variant, "State"=enum."Pause"} ("Data"), error in (no error)=w792) -> (error out=w799:errorcluster)  [unwired: 1 in, 2 out]
            n138 = call "JL_Get_Latest_Build_From_Artifactory.vi"("Repository"="CIBuild") -> ("Output Path"=w786:path)  [unwired: 12 in, 2 out]
            n139 = call "Time Delay2"("error in (no error)"=w799, "Delay Time (s)"=3.0) -> ("error out"=w798:errorcluster)  [unwired: 9 in]
            n140 = Not Equal?(x=w786, y=path "") -> (x != y?=w804:bool)
            n141 = case shown="True" w804 {
              tunnel: w798 -> [w807 w831]
              tunnel: [w807 w819] -> w789
              tunnel: w802 -> [_ w832]
              tunnel: w786 -> [_ w808]
              frame False {
              }
              frame True {
                w811 = T8 9 items=["ImageRejected", "BoardNotFound", "UnableToGetGeaConfiguration", "WriteToFlashNotAllowed", "ImageDownloadedSuccessfully", "ImagePresent", "WriteToFlashFailed", "EraseFailed", "CrcFailed", ""] ("Result")
                w818 = FALSE ("Blinking")
                n142 = call "JL_APLPath.vi"("Error In"=w831, "APL Search String"=T43."UI Application APL", "Folder Path"=w808) -> ("Error Out"=w830:errorcluster, "File Path"=w829:path)  [unwired: 5 in, 2 out]
                n143 = call "GEA2 Flash APL.vi"("GEA2 Reference In"=w832, "Force Update?"=TRUE, "Source Address"=u8 228, "Destination Address"=u8 36, "File Path"=w829, "Error In"=w830, "Broadcast"=TRUE, "Reset?"=FALSE ("Reset Board?")) -> ("GEA2 Reference Out"=w821:refnum<k24>, "Result"=w815:i32, "Error Out"=w817:errorcluster)  [unwired: 3 in, 2 out]
                n144 = property on="Board Index" class="DigNum (strict)"(error in=w831, "DisabledEnum"=T41."Disabled and Grayed Out" ("Disabled")) -> (error out=w814:errorcluster)  [unwired: 1 in, 1 out]
                n145 = property on="Result" class="Ring (strict)"(error in=w817, "Value"=w815) -> (error out=w816:errorcluster)  [unwired: 1 in, 1 out]
                n146 = property on="Result" class="Ring (strict)"(error in=w814, "Value"=w811) -> ()  [unwired: 1 in, 2 out]
                n147 = call "JL_APLPath.vi"("Error In"=w816, "APL Search String"=T43."UI Parametric APL", "Folder Path"=w808) -> ("Error Out"=w827:errorcluster, "File Path"=w828:path)  [unwired: 5 in, 2 out]
                n148 = call "GEA2 Flash APL.vi"("GEA2 Reference In"=w821, "Force Update?"=TRUE, "Source Address"=u8 228, "Destination Address"=u8 36, "File Path"=w828, "Error In"=w827, "Broadcast"=TRUE, "Reset?"=TRUE ("Reset Board?")) -> ("Result"=w812:i32, "Error Out"=w820:errorcluster)  [unwired: 3 in, 3 out]
                n149 = property on="Board Index" class="DigNum (strict)"(error in=w820, "DisabledEnum"=T41."Enabled" ("Disabled")) -> (error out=w813:errorcluster)  [unwired: 1 in, 1 out]
                n150 = property on="Program Ind" class="Bool (strict)"(error in=w820, "Value"=w818, "Blinking"=w818) -> (error out=w819:errorcluster)  [unwired: 1 in, 1 out]
                n151 = property on="Result" class="Ring (strict)"(error in=w813, "Value"=w812) -> ()  [unwired: 1 in, 2 out]
              }
            }
            n152 = call "Time Delay4"("error in (no error)"=w789, "Delay Time (s)"=3.0) -> ("error out"=w788:errorcluster)  [unwired: 9 in]
            n153 = Enqueue Element(queue=w797, element=T37 {"Data"=variant, "State"=enum."Init"} ("Data"), error in (no error)=w788) -> (error out=w796:errorcluster)  [unwired: 1 in, 2 out]
          }
          event Value Change {
            n154 = event-data() -> ()  [unwired: 1 in, 6 out]
            n155 = property on="GEA2 Send" class="Clust (strict)"() -> ("Value"=w843:T9)  [unwired: 2 in, 2 out]
            n156 = Unbundle By Name(w843) -> ("Source"=w842:u8)
            n157 = Bundle By Name(cluster=T9 {"Source"=228, "Destination"=36, "Command"=221, "Message"="F401"} ("Input Data"), "Source"=w842, "Destination"=u8 255, "Command"=u8 221, "Message"="F401") -> (w846:T9)
            n158 = call "GEA2 Send Message.vi"("GEA2 Reference In"=w853, "Input Data"=w846, "Error In"=w854) -> ("Error Out"=w840:errorcluster)  [unwired: 11 in, 1 out]
            n159 = call "Time Delay5"("error in (no error)"=w840, "Delay Time (s)"=3.0) -> ("error out"=w850:errorcluster)  [unwired: 9 in]
            n160 = Enqueue Element(queue=w848, element=T37 {"Data"=variant, "State"=enum."Init"} ("Data"), error in (no error)=w850) -> (error out=w849:errorcluster)  [unwired: 1 in, 2 out]
          }
          event Value Change {
            n161 = event-data() -> ()  [unwired: 1 in, 6 out]
            n162 = property on="GEA2 Send" class="Clust (strict)"() -> ("Value"=w862:T9)  [unwired: 2 in, 2 out]
            n163 = Unbundle By Name(w862) -> ("Source"=w858:u8, "Destination"=w857:u8)
            n164 = Bundle By Name(cluster=T9 {"Source"=228, "Destination"=36, "Command"=221, "Message"="F401"} ("Input Data"), "Source"=w858, "Destination"=w857, "Command"=u8 221, "Message"="07") -> (w856:T9)
            n165 = call "GEA2 Send Message.vi"("GEA2 Reference In"=w864, "Input Data"=w856, "Error In"=w865) -> ("GEA2 Reference Out"=w863:refnum<k24>, "Error Out"=w855:errorcluster)  [unwired: 11 in]
          }
          event Value Change {
            n166 = event-data() -> ("CtlRef"=w874:refnum<vi>)  [unwired: 1 in, 5 out]
            n167 = property class="Bool"(reference=w874, error in=w872) -> (error out=w871:errorcluster, "Label.Text"=w873:string)  [unwired: 1 out]
            n168 = case shown="\"Relays ON\"" w873 {
              tunnel: w871 -> [w888 w909]
              tunnel: [w887 w916] -> w870
              tunnel: "Relay Control" -> [w901 _]
              tunnel: w868 -> [w886 w915]
              tunnel: [w881 w911] -> w867
              tunnel: w866 -> [w876 w903]
              frame "Relays ON" {
                n169 = Unbundle By Name(w901) -> ("Drum Motor"=w898:bool, "HTR 1 / Inner / Top"=w893:bool, "HTR 2 / Outer / Bot"=w892:bool, "Steam Valve"=w891:bool)
                n170 = Boolean To (0,1)(Boolean=w898) -> (0, 1=w900:i16)
                n171 = Boolean To (0,1)(Boolean=w893) -> (0, 1=w897:i16)
                n172 = Boolean To (0,1)(Boolean=w892) -> (0, 1=w895:i16)
                n173 = Boolean To (0,1)(Boolean=w891) -> (0, 1=w894:i16)
                n174 = Number To Hexadecimal String(1:i16 2 ("width (-)"), 2:w900) -> (0:w899:string)
                n175 = Number To Hexadecimal String(1:i16 2 ("width (-)"), 2:w897) -> (0:w896:string)
                n176 = Number To Hexadecimal String(1:i16 2 ("width (-)"), 2:w895) -> (0:w890:string)
                n177 = Number To Hexadecimal String(1:i16 2 ("width (-)"), 2:w894) -> (0:w889:string)
                n178 = Concatenate Strings(w899, w896, w890, w889) -> (w884:string)
                n179 = Bundle By Name(cluster=T42 {"ERD Number"=62208, "Data Type"=enum."string", "Data"=""} ("ERD Read Data In"), "Data"=w884) -> (w883:T42)
                n180 = Build Array(w883) -> (w882:T42[])
                n181 = call "GEA2 Write ERD.vi"("GEA2 Reference In"=w886, "GEA Inputs"=w876, "Write ERD List"=w882, "Error In"=w888, "Verify ERD Response?"=TRUE) -> ("GEA2 Reference Out"=w881:refnum<k24>, "Error Out"=w887:errorcluster)  [unwired: 8 in, 1 out]
              }
              frame "Relays OFF", Default {
                w904 = FALSE ("Value")
                n182 = property on="Drum Motor" class="Bool (strict)"(error in=w909, "Value"=w904) -> (error out=w908:errorcluster)  [unwired: 1 in, 1 out]
                n183 = property on="HTR 1 / Inner / Top" class="Bool (strict)"(error in=w908, "Value"=w904) -> (error out=w907:errorcluster)  [unwired: 1 in, 1 out]
                n184 = property on="HTR 2 / Outer / Bot" class="Bool (strict)"(error in=w907, "Value"=w904) -> (error out=w906:errorcluster)  [unwired: 1 in, 1 out]
                n185 = property on="Steam Valve" class="Bool (strict)"(error in=w906, "Value"=w904) -> (error out=w905:errorcluster)  [unwired: 1 in, 1 out]
                n186 = Bundle By Name(cluster=T42 {"ERD Number"=62208, "Data Type"=enum."string", "Data"=""} ("ERD Read Data In"), "Data"="00000000") -> (w913:T42)
                n187 = Build Array(w913) -> (w912:T42[])
                n188 = call "GEA2 Write ERD.vi"("GEA2 Reference In"=w915, "GEA Inputs"=w903, "Write ERD List"=w912, "Error In"=w905, "Verify ERD Response?"=TRUE) -> ("GEA2 Reference Out"=w911:refnum<k24>, "Error Out"=w916:errorcluster)  [unwired: 8 in, 1 out]
              }
            }
          }
          event Value Change {
            n189 = event-data() -> ("CtlRef"=w925:refnum<vi>)  [unwired: 1 in, 5 out]
            n190 = property class="Ctl"(reference=w925, error in=w923) -> (error out=w922:errorcluster, "Label.Text"=w924:string)  [unwired: 1 out]
            n191 = case shown="\"Drum Light OFF\", Default" w924 {
              tunnel: w922 -> [w929 w940 w954]
              tunnel: [w932 w939 w953] -> w921
              tunnel: "Drum Light" -> [_ _ w948]
              tunnel: w920 -> [w928 w938 w952]
              tunnel: [w930 w935 w951] -> w919
              tunnel: w918 -> [w926 w934 w950]
              frame "Drum Light ON" {
                n192 = Build Array(T42 {"ERD Number"=61582, "Data Type"=enum."string", "Data"="01"} ("ERD Read Data In")) -> (w927:T42[])
                n193 = call "GEA2 Write ERD.vi"("GEA2 Reference In"=w928, "GEA Inputs"=w926, "Write ERD List"=w927, "Error In"=w929) -> ("GEA2 Reference Out"=w930:refnum<k24>, "Error Out"=w932:errorcluster)  [unwired: 9 in, 1 out]
              }
              frame "Drum Light OFF", Default {
                n194 = Build Array(T42 {"ERD Number"=61582, "Data Type"=enum."string", "Data"="00"} ("ERD Read Data In")) -> (w936:T42[])
                n195 = call "GEA2 Write ERD.vi"("GEA2 Reference In"=w938, "GEA Inputs"=w934, "Write ERD List"=w936, "Error In"=w940, "Verify ERD Response?"=TRUE) -> ("GEA2 Reference Out"=w935:refnum<k24>, "Error Out"=w939:errorcluster)  [unwired: 8 in, 1 out]
              }
              frame "On Time (s)" {
                n196 = Unbundle By Name(w948) -> ("On Time (s)"=w945:dbl)
                n197 = Multiply(x=w945, y=1000.0) -> (x*y=w943:dbl)
                n198 = Number To Decimal String(number=w943) -> (decimal integer string=w942:string)  [unwired: 1 in]
                n199 = Bundle By Name(cluster=T42 {"ERD Number"=61482, "Data Type"=enum."uint32_t", "Data"=""} ("ERD Read Data In"), "Data"=w942) -> (w947:T42)
                n200 = Build Array(w947) -> (w946:T42[])
                n201 = call "GEA2 Write ERD.vi"("GEA2 Reference In"=w952, "GEA Inputs"=w950, "Write ERD List"=w946, "Error In"=w954, "Verify ERD Response?"=TRUE) -> ("GEA2 Reference Out"=w951:refnum<k24>, "Error Out"=w953:errorcluster)  [unwired: 8 in, 1 out]
              }
            }
          }
          event "Reset": Value Change {
            n202 = event-data() -> ()  [unwired: 1 in, 6 out]
            n203 = call "Convert Write ERD List to Message.vi"("GEA Inputs"=w959, "Write ERD List"=T42[] [{"ERD Number"=50, "Data Type"=enum."string", "Data"="01"}], "Error In"=w964) -> ("Error Out"=w955:errorcluster)  [unwired: 11 in, 1 out]
            n204 = call "Reset Board.vi"("GEA2 Reference In"=w957, "Error In"=w955) -> ("GEA2 Reference Out"=w956:refnum<k24>, "Error Out"=w958:errorcluster)  [unwired: 10 in, 2 out]
            n205 = Enqueue Element(queue=w961, element=T37 {"Data"=variant, "State"=enum."Init"} ("Data"), error in (no error)=w958) -> (error out=w962:errorcluster)  [unwired: 1 in, 2 out]
          }
          event "Save Log": Value Change {
            n206 = event-data() -> ()  [unwired: 1 in, 6 out]
            n207 = property on="GEA2 Log" class="Str"(error in=w970) -> (error out=w972:errorcluster, "Value"=w971:string)  [unwired: 1 in, 1 out]
            n208 = Write to Text File(prompt (Choose or enter file path)="Choose filename and path to save txt file to ", text=w971, error in=w972) -> (refnum out=w969:refnum<file>, error out=w968:errorcluster)  [unwired: 1 in, 1 out]
            n209 = Close File(refnum=w969, error in=w968) -> (error out=w967:errorcluster)  [unwired: 1 out]
            n210 = call <vilib>:"Clear Errors.vi"("error in (no error)"=w967, "specific error code to clear (0: all)"=43) -> ("error out"=w966:errorcluster)  [unwired: 4 in, 1 out]
          }
          event "Desired FilteredMoisture": Value Change {
            n211 = event-data() -> ()  [unwired: 1 in, 6 out]
            n212 = call "MoistureSensorReset.vi"("GEA2 Reference In"=w975, "Error In"=w977) -> ("Error Out"=w974:errorcluster)  [unwired: 10 in, 3 out]
            n213 = call "JL_Scaling Factor.vi"("Error"=w974, "Scalling"="Scalling", "Scaling Type"="Init/Scale", "Desired Value Out"="Desired FilteredMoisture") -> ("Error Out"=w976:errorcluster, "Analog Value Out"=w981:dbl)  [unwired: 5 in, 1 out]
            n214 = property on="Moisture (V)" class="Slide (strict)"("Value"=w981) -> ()  [unwired: 2 in, 2 out]
          }
          event "Model": Value Change {
            n215 = event-data() -> ("NewVal"=w984:enum16{"Estar Centauro", "GFL"})  [unwired: 1 in, 5 out]
            n216 = call "Set Get Model.vi"("Error In"=w982, "Action"=enum16{"Set Model", "Get Model"}."Set Model", "Model"=w984) -> ()  [unwired: 7 in, 2 out]
          }
          event "Run Script": Value Change {
            w1012 = T32 {"Overall Script File Progress"=0.0, "Current Script Progress"=0.0, "Script"="", "Test"="", "Elapsed time (s)"=0.0, "Done?"=FALSE}  # Script Info
            w1004 = T9 {"Source"=228, "Destination"=35, "Command"=1, "Message"=""}  # Version Query (for log header)
            n217 = event-data() -> ()  [unwired: 1 in, 6 out]
            n218 = Generate User Event(user event=w985, event data cluster=TRUE ("event data"), error in=w988) -> (error out=w989:errorcluster)  [unwired: 1 in, 1 out]
            n219 = Enqueue Element(queue=w986, element=T37 {"Data"=variant, "State"=enum."Pause"} ("Data"), error in (no error)=w989) -> (error out=w987:errorcluster)  [unwired: 1 in, 2 out]
            n220 = Obtain Queue(name (unnamed)="Script_Stop", element data type=FALSE, error in (no error)=w987) -> (queue out=w1008:refnum<queue>, error out=w1011:errorcluster)  [unwired: 2 in, 1 out]
            n221 = Obtain Queue(name (unnamed)="Script_Info", element data type=w1012, error in (no error)=w1011) -> (queue out=w1014:refnum<queue>, error out=w1005:errorcluster)  [unwired: 2 in, 1 out]
            n222 = while {
              tunnel: w1014 -> [w1026]
              shift-right: [w1019] -> w1002
              shift-left: w1005 -> [w1022]
              tunnel: [w1025] -> w1013
              tunnel: w1008 -> [w1023]
              tunnel: [w1018] -> w1006
              stop <- w1024 stop-if-true
              n223 = Dequeue Element(queue=w1026, error in (no error)=w1022) -> (queue out=w1025:refnum<queue>, element=w1017:T32, error out=w1021:errorcluster)  [unwired: 1 in, 1 out]
              "Script Info" <- w1017
              n224 = Unbundle By Name(w1017) -> ("Done?"=w1024:bool)
              n225 = case shown="False" "stop script" {
                selector: "stop script" -> [_ w1029]
                tunnel: w1023 -> [w1028 w1033]
                tunnel: w1022 -> [w1027 w1032]
                tunnel: [w1027 w1031] -> w1020
                tunnel: [w1028 w1030] -> w1018
                frame False {
                }
                frame True {
                  n226 = Enqueue Element(queue=w1033, element=w1029, error in (no error)=w1032) -> (queue out=w1030:refnum<queue>, error out=w1031:errorcluster)  [unwired: 1 in, 1 out]
                }
              }
              n227 = Merge Errors(w1020, w1021) -> (w1019:errorcluster)
            }
            n228 = call "GEA2 Script Test SLB.vi"("GEA2 Reference In"=w1000, "Version Query (for log header)"=w1004, "Enqueue Sends?"=TRUE, "Standalone"=FALSE, "Script path"="Script Path", "Log File Path (empty for prompt)"="Script Log Path", "Error In"=w1005) -> ("Pass/Fail?"=→"Script Pass/Fail?":bool, "Report Text"=→"Script Report Text":string, "Error Out"=→"Script Error Out":errorcluster)  [unwired: 5 in, 1 out]
            n229 = Release Queue(queue=w1013, error in (no error)=w1002) -> (error out=w1007:errorcluster)  [unwired: 1 in, 2 out]
            n230 = Release Queue(queue=w1006, error in (no error)=w1007) -> (error out=w992:errorcluster)  [unwired: 1 in, 2 out]
            n231 = Enqueue Element(queue=w986, element=T37 {"Data"=variant, "State"=enum."Init"} ("Data"), error in (no error)=w992) -> (error out=w991:errorcluster)  [unwired: 1 in, 2 out]
          }
          event Value Change {
            n232 = event-data() -> ("CtlRef"=w1036:refnum<vi>)  [unwired: 1 in, 5 out]
            n233 = property class="Bool"(reference=w1036, error in=w1037) -> (reference out=w1041:refnum<vi>, error out=w1042:errorcluster, "Label.Text"=w1040:string)
            n234 = Close Reference(reference=w1041, error in (no error)=w1042) -> (error out=w1043:errorcluster)
            n235 = case shown="\"Pause Cycle\"" w1040 {
              tunnel: w1043 -> [w1050 w1066 w1082 w1098 w1114]
              tunnel: w1039 -> [w1051 w1067 w1083 w1099 w1115]
              tunnel: w1038 -> [w1049 w1065 w1081 w1097 w1113]
              tunnel: [w1046 w1062 w1078 w1094 w1110] -> w1034
              tunnel: [w1048 w1064 w1080 w1096 w1112] -> w1035
              frame "Start Cycle" {
                n236 = property on="Cycle Selection" class="DigNum (strict)"(error in=w1050) -> (error out=w1044:errorcluster, "Value"=w1047:u8)  [unwired: 1 in, 1 out]
                n237 = Number To Hexadecimal String(1:i16 2 ("width (-)"), 2:w1047) -> (0:w1059:string)
                n238 = Concatenate Strings("01" ("string"), w1059, "01" ("string")) -> (w1057:string)
                n239 = Bundle By Name(cluster=T42 {"ERD Number"=62720, "Data Type"=enum."string", "Data"=""} ("ERD Read Data In"), "Data"=w1057) -> (w1055:T42)
                n240 = Build Array(w1055) -> (w1053:T42[])
                n241 = call "GEA2 Write ERD.vi"("GEA2 Reference In"=w1049, "GEA Inputs"=w1051, "Write ERD List"=w1053, "Error In"=w1044, "Verify ERD Response?"=TRUE) -> ("GEA2 Reference Out"=w1046:refnum<k24>, "Error Out"=w1048:errorcluster)  [unwired: 8 in, 1 out]
              }
              frame "Stop Cycle", Default {
                n242 = property on="Cycle Selection" class="DigNum (strict)"(error in=w1066) -> (error out=w1060:errorcluster, "Value"=w1063:u8)  [unwired: 1 in, 1 out]
                n243 = Number To Hexadecimal String(1:i16 2 ("width (-)"), 2:w1063) -> (0:w1075:string)
                n244 = Concatenate Strings("01" ("string"), w1075, "02" ("string")) -> (w1073:string)
                n245 = Bundle By Name(cluster=T42 {"ERD Number"=62720, "Data Type"=enum."string", "Data"=""} ("ERD Read Data In"), "Data"=w1073) -> (w1071:T42)
                n246 = Build Array(w1071) -> (w1069:T42[])
                n247 = call "GEA2 Write ERD.vi"("GEA2 Reference In"=w1065, "GEA Inputs"=w1067, "Write ERD List"=w1069, "Error In"=w1060, "Verify ERD Response?"=TRUE) -> ("GEA2 Reference Out"=w1062:refnum<k24>, "Error Out"=w1064:errorcluster)  [unwired: 8 in, 1 out]
              }
              frame "Pause Cycle" {
                n248 = property on="Cycle Selection" class="DigNum (strict)"(error in=w1082) -> (error out=w1076:errorcluster, "Value"=w1079:u8)  [unwired: 1 in, 1 out]
                n249 = Number To Hexadecimal String(1:i16 2 ("width (-)"), 2:w1079) -> (0:w1091:string)
                n250 = Concatenate Strings("01" ("string"), w1091, "03" ("string")) -> (w1089:string)
                n251 = Bundle By Name(cluster=T42 {"ERD Number"=62720, "Data Type"=enum."string", "Data"=""} ("ERD Read Data In"), "Data"=w1089) -> (w1087:T42)
                n252 = Build Array(w1087) -> (w1085:T42[])
                n253 = call "GEA2 Write ERD.vi"("GEA2 Reference In"=w1081, "GEA Inputs"=w1083, "Write ERD List"=w1085, "Error In"=w1076, "Verify ERD Response?"=TRUE) -> ("GEA2 Reference Out"=w1078:refnum<k24>, "Error Out"=w1080:errorcluster)  [unwired: 8 in, 1 out]
              }
              frame "Resume Cycle" {
                n254 = property on="Cycle Selection" class="DigNum (strict)"(error in=w1098) -> (error out=w1092:errorcluster, "Value"=w1095:u8)  [unwired: 1 in, 1 out]
                n255 = Number To Hexadecimal String(1:i16 2 ("width (-)"), 2:w1095) -> (0:w1107:string)
                n256 = Concatenate Strings("01" ("string"), w1107, "04" ("string")) -> (w1105:string)
                n257 = Bundle By Name(cluster=T42 {"ERD Number"=62720, "Data Type"=enum."string", "Data"=""} ("ERD Read Data In"), "Data"=w1105) -> (w1103:T42)
                n258 = Build Array(w1103) -> (w1101:T42[])
                n259 = call "GEA2 Write ERD.vi"("GEA2 Reference In"=w1097, "GEA Inputs"=w1099, "Write ERD List"=w1101, "Error In"=w1092, "Verify ERD Response?"=TRUE) -> ("GEA2 Reference Out"=w1094:refnum<k24>, "Error Out"=w1096:errorcluster)  [unwired: 8 in, 1 out]
              }
              frame "Select Cycle" {
                n260 = property on="Cycle Selection" class="DigNum (strict)"(error in=w1114) -> (error out=w1108:errorcluster, "Value"=w1111:u8)  [unwired: 1 in, 1 out]
                n261 = Number To Hexadecimal String(1:i16 2 ("width (-)"), 2:w1111) -> (0:w1123:string)
                n262 = Concatenate Strings("01" ("string"), w1123, "05" ("string")) -> (w1121:string)
                n263 = Bundle By Name(cluster=T42 {"ERD Number"=62720, "Data Type"=enum."string", "Data"=""} ("ERD Read Data In"), "Data"=w1121) -> (w1119:T42)
                n264 = Build Array(w1119) -> (w1117:T42[])
                n265 = call "GEA2 Write ERD.vi"("GEA2 Reference In"=w1113, "GEA Inputs"=w1115, "Write ERD List"=w1117, "Error In"=w1108, "Verify ERD Response?"=TRUE) -> ("GEA2 Reference Out"=w1110:refnum<k24>, "Error Out"=w1112:errorcluster)  [unwired: 8 in, 1 out]
              }
            }
          }
          event "LED Control.ALL LEDs ON", "LED Control.ALL LEDs OFF", "LED Control.Reset LEDs": Value Change {
            n266 = event-data() -> ("CtlRef"=w1126:refnum<vi>)  [unwired: 1 in, 5 out]
            n267 = property class="Bool"(reference=w1126, error in=w1127) -> (reference out=w1131:refnum<vi>, error out=w1132:errorcluster, "Label.Text"=w1130:string)
            n268 = Close Reference(reference=w1131, error in (no error)=w1132) -> (error out=w1133:errorcluster)
            n269 = case shown="\"Reset LEDS\", Default" w1130 {
              tunnel: w1133 -> [w1138 w1155 w1174]
              tunnel: w1129 -> [w1139 w1156 w1172]
              tunnel: w1128 -> [w1137 w1154 w1173]
              tunnel: [w1136 w1153 w1171] -> w1124
              tunnel: [w1135 w1152 w1170] -> w1125
              frame "ALL LEDs ON" {
                n270 = Concatenate Strings("0101FFFFFFFFFFFFFFFFFFFF" ("string")) -> (w1150:string)
                n271 = Bundle By Name(cluster=T42 {"ERD Number"=61724, "Data Type"=enum."string", "Data"=""} ("ERD Read Data In"), "Data"=w1150) -> (w1148:T42)
                n272 = Build Array(w1148) -> (w1141:T42[])
                n273 = call "Convert Write ERD List to Message.vi"("GEA Inputs"=w1139, "Write ERD List"=w1141, "Error In"=w1138) -> ("GEA Message"=w1143:T9, "Error Out"=w1144:errorcluster)  [unwired: 11 in]
                n274 = call "GEA2MessageFormatter.vi"("Prefix(Send/Recv)"="SEND", "GEA2 Data In"=w1143, "Error In"=w1144) -> ("Output String"=w1145:string, "Error Out"=w1146:errorcluster)  [unwired: 11 in]
                n275 = call "GExplorer_Queue_GEA2.vi"("Output String"=w1145, "error in (no error)"=w1146) -> ("error out"=w1142:errorcluster)  [unwired: 13 in]
                n276 = call "GEA2 Write ERD.vi"("GEA2 Reference In"=w1137, "GEA Inputs"=w1139, "Write ERD List"=w1141, "Error In"=w1142, "Verify ERD Response?"=TRUE) -> ("GEA2 Reference Out"=w1136:refnum<k24>, "Error Out"=w1135:errorcluster)  [unwired: 8 in, 1 out]
              }
              frame "ALL LEDs OFF" {
                n277 = Concatenate Strings("010100000000000000000000" ("string")) -> (w1167:string)
                n278 = Bundle By Name(cluster=T42 {"ERD Number"=61724, "Data Type"=enum."string", "Data"=""} ("ERD Read Data In"), "Data"=w1167) -> (w1165:T42)
                n279 = Build Array(w1165) -> (w1158:T42[])
                n280 = call "Convert Write ERD List to Message.vi"("GEA Inputs"=w1156, "Write ERD List"=w1158, "Error In"=w1155) -> ("GEA Message"=w1160:T9, "Error Out"=w1161:errorcluster)  [unwired: 11 in]
                n281 = call "GEA2MessageFormatter.vi"("Prefix(Send/Recv)"="SEND", "GEA2 Data In"=w1160, "Error In"=w1161) -> ("Output String"=w1162:string, "Error Out"=w1163:errorcluster)  [unwired: 11 in]
                n282 = call "GExplorer_Queue_GEA2.vi"("Output String"=w1162, "error in (no error)"=w1163) -> ("error out"=w1159:errorcluster)  [unwired: 13 in]
                n283 = call "GEA2 Write ERD.vi"("GEA2 Reference In"=w1154, "GEA Inputs"=w1156, "Write ERD List"=w1158, "Error In"=w1159, "Verify ERD Response?"=TRUE) -> ("GEA2 Reference Out"=w1153:refnum<k24>, "Error Out"=w1152:errorcluster)  [unwired: 8 in, 1 out]
              }
              frame "Reset LEDS", Default {
                n284 = Concatenate Strings("010100000000000000000000" ("string")) -> (w1187:string)
                n285 = Bundle By Name(cluster=T42 {"ERD Number"=61724, "Data Type"=enum."string", "Data"=""} ("ERD Read Data In"), "Data"=w1187) -> (w1185:T42)
                n286 = Build Array(w1185) -> (w1178:T42[])
                n287 = call "Convert Write ERD List to Message.vi"("GEA Inputs"=w1172, "Write ERD List"=w1178, "Error In"=w1174) -> ("GEA Message"=w1180:T9, "Error Out"=w1181:errorcluster)  [unwired: 11 in]
                n288 = call "GEA2MessageFormatter.vi"("Prefix(Send/Recv)"="SEND", "GEA2 Data In"=w1180, "Error In"=w1181) -> ("Output String"=w1182:string, "Error Out"=w1183:errorcluster)  [unwired: 11 in]
                n289 = call "GExplorer_Queue_GEA2.vi"("Output String"=w1182, "error in (no error)"=w1183) -> ("error out"=w1179:errorcluster)  [unwired: 13 in]
                n290 = call "GEA2 Write ERD.vi"("GEA2 Reference In"=w1173, "GEA Inputs"=w1172, "Write ERD List"=w1178, "Error In"=w1179, "Verify ERD Response?"=TRUE) -> ("GEA2 Reference Out"=w1175:refnum<k24>, "Error Out"=w1176:errorcluster)  [unwired: 8 in, 1 out]
                n291 = Concatenate Strings("000000000000000000000000" ("string")) -> (w1198:string)
                n292 = Bundle By Name(cluster=T42 {"ERD Number"=61724, "Data Type"=enum."string", "Data"=""} ("ERD Read Data In"), "Data"=w1198) -> (w1196:T42)
                n293 = Build Array(w1196) -> (w1189:T42[])
                n294 = call "Convert Write ERD List to Message.vi"("GEA Inputs"=w1172, "Write ERD List"=w1189, "Error In"=w1176) -> ("GEA Message"=w1191:T9, "Error Out"=w1192:errorcluster)  [unwired: 11 in]
                n295 = call "GEA2MessageFormatter.vi"("Prefix(Send/Recv)"="SEND", "GEA2 Data In"=w1191, "Error In"=w1192) -> ("Output String"=w1193:string, "Error Out"=w1194:errorcluster)  [unwired: 11 in]
                n296 = call "GExplorer_Queue_GEA2.vi"("Output String"=w1193, "error in (no error)"=w1194) -> ("error out"=w1190:errorcluster)  [unwired: 13 in]
                n297 = call "GEA2 Write ERD.vi"("GEA2 Reference In"=w1175, "GEA Inputs"=w1172, "Write ERD List"=w1189, "Error In"=w1190, "Verify ERD Response?"=TRUE) -> ("GEA2 Reference Out"=w1171:refnum<k24>, "Error Out"=w1170:errorcluster)  [unwired: 8 in, 1 out]
              }
            }
          }
          event Value Change {
            n298 = event-data() -> ()  [unwired: 1 in, 6 out]
            n299 = Enqueue Element(queue=w1202, element=T37 {"Data"=variant, "State"=enum."Build ERD Read List"}, error in (no error)=w1204) -> (error out=w1203:errorcluster)  [unwired: 1 in, 2 out]
            n300 = call "Select_List.vi"("Load ERD List"="Load ERD List") -> ("ERD Read List"=w1199:T33)  [unwired: 14 in]
            n301 = call "Write_Header_FGV.vi"("Write Header ? In"=TRUE, "Action"=enum16{"Get", "Set"}."Set", "Error In"=w1203) -> ("Error Out"=w1206:errorcluster)  [unwired: 11 in, 1 out]
            n302 = property on="ERD Read List" class="Arr (strict)"("Value"=w1199) -> ()  [unwired: 2 in, 2 out]
          }
          event "Clear Fault Seq Buffer": Value Change {
            n303 = event-data() -> ()  [unwired: 1 in, 6 out]
            n304 = Bundle By Name(cluster=T42 {"ERD Number"=57626, "Data Type"=enum."string", "Data"=""} ("ERD Read Data In"), "Data"="01") -> (w1221:T42)
            n305 = Build Array(w1221) -> (w1215:T42[])
            n306 = call "Convert Write ERD List to Message.vi"("GEA Inputs"=w1212, "Write ERD List"=w1215, "Error In"=w1211) -> ("GEA Message"=w1217:T9, "Error Out"=w1218:errorcluster)  [unwired: 11 in]
            n307 = call "GEA2MessageFormatter.vi"("Prefix(Send/Recv)"="SEND", "GEA2 Data In"=w1217, "Error In"=w1218) -> ("Output String"=w1219:string, "Error Out"=w1220:errorcluster)  [unwired: 11 in]
            n308 = call "GExplorer_Queue_GEA2.vi"("Output String"=w1219, "error in (no error)"=w1220) -> ("error out"=w1216:errorcluster)  [unwired: 13 in]
            n309 = call "GEA2 Write ERD.vi"("GEA2 Reference In"=w1210, "GEA Inputs"=w1212, "Write ERD List"=w1215, "Error In"=w1216) -> ("GEA2 Reference Out"=w1209:refnum<k24>, "Error Out"=w1208:errorcluster)  [unwired: 9 in, 1 out]
          }
          event "Get Faults": Value Change {
            n310 = event-data() -> ()  [unwired: 1 in, 6 out]
            n311 = call "Main_Decode_V3.vi"("GEA2 Reference In"=w1226, "GEA Inputs"=w1230, "Error In"=w1229) -> ("Fault Table Status"=w1248:T20[], "Major Version"=→"Major Version":u8, "Minor Version"=→"Minor Version":u8, "Fault Table Entries"=w1247:T21[][], "GEA2 Reference Out"=w1237:refnum<k24>, "Diagnostic Entity Manifest"=w1245:T22[], "SnapShot ERD List"=w1235:T12[][], "Fault Sequence Status"=w1238:T20[], "Fault Sequence Entries"=w1246:T19[][], "Error Out"=w1236:errorcluster)  [unwired: 5 in, 2 out]
            n312 = Index Array(array=w1247) -> (element=w1243:T21[])  [unwired: 2 in]
            n313 = Index Array(array=w1248) -> (element=w1224:T20)  [unwired: 1 in]
            "Fault Table Status" <- w1224
            n314 = Index Array(array=w1245) -> (element=→"Diagnostic Entity Manifest":T22)  [unwired: 1 in]
            n315 = Index Array(array=w1246) -> (element=w1240:T19[])  [unwired: 2 in]
            n316 = Index Array(array=w1238) -> (element=w1233:T20)  [unwired: 1 in]
            "Fault Seq Status" <- w1233
            n317 = call "JL_Diag_Filter_Faults.vi"("Filter by Count"="Filter by Count", "Fault Table Entries In"=w1243, "Status"=w1224) -> ("Fault Table Entries Out"=→"Fault Table Entries":T21[], "Fault Set?"=→"Fault Set?":bool)  [unwired: 11 in]
            n318 = call "JL_Diag_Filter_Seq.vi"("Filter by Count"="Filter by Count", "Fault Table Entries In"=w1240, "Status"=w1233) -> ("Fault Table Entries Out"=→"Fault Sequence Entries":T19[])  [unwired: 12 in]
            n319 = Unbundle By Name(w1224) -> ("Count"=w1223:u16)
            n320 = Index Array(array=w1235) -> (element=w1234:T12[])  [unwired: 2 in]
            n321 = for {
              N: w1223 -> [_]
              tunnel: [w1257] -> w1232 mode=indexing
              tunnel: w1230 -> [w1255]
              shift-right: [w1254] -> w1227
              shift-left: w1237 -> [w1256]
              shift-right: [w1252] -> w1228
              shift-left: w1236 -> [w1253]
              tunnel: w1234 -> [w1251] mode=indexing
              tunnel: "Filter by Count" -> [_]
              n322 = call "JL_Parse_Snapshot.vi"("GEA2 Reference In"=w1256, "GEA Inputs"=w1255, "SnapShot Location"=w1251, "Error In"=w1253) -> ("GEA2 Reference Out"=w1254:refnum<k24>, "Fault Snapshot"=w1257:string[], "Error Out"=w1252:errorcluster)  [unwired: 9 in]
            }
            n323 = Transpose 2D Array(2D array=w1232) -> (transposed array=→"Centauro Fault Snapshot":string[][])
          }
          event "Clear Fault Table Buffer": Value Change {
            n324 = event-data() -> ()  [unwired: 1 in, 6 out]
            n325 = Bundle By Name(cluster=T42 {"ERD Number"=57604, "Data Type"=enum."string", "Data"=""} ("ERD Read Data In"), "Data"="01") -> (w1265:T42)
            n326 = Build Array(w1265) -> (w1264:T42[])
            n327 = call "GEA2 Write ERD.vi"("GEA2 Reference In"=w1261, "GEA Inputs"=w1262, "Write ERD List"=w1264, "Error In"=w1258) -> ("GEA2 Reference Out"=w1260:refnum<k24>, "Error Out"=w1259:errorcluster)  [unwired: 9 in, 1 out]
          }
          event "Get Cycle Data": Value Change {
            w1280 = T12[] [{"ERD Number"=57661, "Data Type"=enum."string"}, {"ERD Number"=57662, "Data Type"=enum."string"}, {"ERD Number"=57663, "Data Type"=enum."string"}, {"ERD Number"=57664, "Data Type"=enum."string"}, {"ERD Number"=57665, "Data Type"=enum."string"}, {"ERD Number"=57666, "Data Type"=enum."string"}, {"ERD Number"=57667, "Data Type"=enum."string"}, {"ERD Number"=57668, "Data Type"=enum."string"}, {"ERD Number"=57669, "Data Type"=enum."string"}, {"ERD Number"=57670, "Data Type"=enum."string"}, {"ERD Number"=57671, "Data Type"=enum."string"}, {"ERD Number"=57672, "Data Type"=enum."string"}, {"ERD Number"=57673, "Data Type"=enum."string"}, {"ERD Number"=57674, "Data Type"=enum."string"}, {"ERD Number"=57675, "Data Type"=enum."string"}, {"ERD Number"=57676, "Data Type"=enum."string"}, {"ERD Number"=57677, "Data Type"=enum."string"}, {"ERD Number"=57678, "Data Type"=enum."string"}, {"ERD Number"=57679, "Data Type"=enum."string"}, {"ERD Number"=57680, "Data Type"=enum."string"}] ("Read ERD List")
            # "Erd_DiagnosticsCycleHistorySequenceEntry[0:19]"
            # "Erd_DiagnosticsCycleHistorySequenceStatus"
            n328 = event-data() -> ()  [unwired: 1 in, 6 out]
            n329 = call "GEA2 Read ERD.vi"("GEA2 Reference In"=w1270, "GEA Inputs"=w1273, "Read ERD List"=T12[] [{"ERD Number"=57659, "Data Type"=enum."string"}], "Error In"=w1269) -> ("GEA2 Reference Out"=w1275:refnum<k24>, "ERD Data Out"=w1278:T48[], "Error Out"=w1274:errorcluster)  [unwired: 8 in, 1 out]
            n330 = Index Array(array=w1278) -> (element=w1279:T48)  [unwired: 1 in]
            n331 = Unbundle By Name(w1279) -> ("Data"=w1291:string)
            n332 = call "HexStringToU16.vi"("Input String"=w1291, "Starting Offset"=0) -> ("Number Out"=w1288:u16)  [unwired: 13 in]
            n333 = call "HexStringToU16.vi"("Input String"=w1291, "Starting Offset"=6) -> ("Number Out"=w1292:u16)  [unwired: 13 in]
            n334 = call "HexStringToU16.vi"("Input String"=w1291, "Starting Offset"=12) -> ("Number Out"=w1289:u16)  [unwired: 13 in]
            n335 = Array Size(array=w1280) -> (size(s)=w1282:i32)
            n336 = Select(t=w1292, s="Filter by Status Count", f=w1282) -> (s? t:f=w1281:i32)
            n337 = Bundle By Name(cluster=T20 {"Cur Index"=0, "Count"=0, "Ov Cnt"=0} ("Fault Table Status"), "Cur Index"=w1288, "Count"=w1292, "Ov Cnt"=w1289) -> (→"Cycle History Status":T20)
            n338 = Array Subset(array=w1280, length=w1281) -> (w1277:T12[])  [unwired: 1 in]
            n339 = for {
              shift-right: [w1298] -> w1272
              shift-left: w1274 -> [w1299]
              shift-right: [w1296] -> w1271
              shift-left: w1275 -> [w1297]
              tunnel: w1277 -> [w1295] mode=indexing
              tunnel: w1273 -> [w1294]
              tunnel: [w1293] -> w1268 mode=indexing
              n340 = call "JL_Cycle_History_ParseRecord.vi"("Error In"=w1299, "Cycle History ERD"=w1295, "GEA Inputs"=w1294, "GEA2 Reference In"=w1297) -> ("Error Out"=w1298:errorcluster, "Centauro CH Record Out"=w1293:string[], "GEA2 Reference Out"=w1296:refnum<k24>)  [unwired: 4 in]
            }
            n341 = Transpose 2D Array(2D array=w1268) -> (transposed array=→"JL Cycle History":string[][])
          }
          event "Data ON": Value Change {
            n342 = event-data() -> ()  [unwired: 1 in, 6 out]
            n343 = case shown="False" "Data ON" {
              tunnel: w1303 -> [w1306 w1310]
              tunnel: [w1305 w1309] -> w1302
              tunnel: w1300 -> [w1304 w1308]
              frame True {
                n344 = Enqueue Element(queue=w1304, element=T37 {"Data"=variant, "State"=enum."Init"} ("Data"), error in (no error)=w1306) -> (error out=w1305:errorcluster)  [unwired: 1 in, 2 out]
              }
              frame False {
                n345 = Enqueue Element(queue=w1308, element=T37 {"Data"=variant, "State"=enum."Pause"} ("Data"), error in (no error)=w1310) -> (error out=w1309:errorcluster)  [unwired: 1 in, 2 out]
              }
            }
          }
          event "Stop": Value Change; User Event; Panel Close {
            n346 = event-data() -> ()  [unwired: 1 in, 3 out]
            n347 = call "Control_ERD_Loop.vi"("Command (ERD Loop Control)"=ERD_Loop_Control_Command."Shutdown", "Error In"=w1320) -> ("Error Out"=w1319:errorcluster)  [unwired: 13 in]
            n348 = call "Control_GEA2_Loop.vi"("Command (ERD Loop Control)"=GEA2_Control_Command."Shutdown", "Error In"=w1319) -> ("Error Out"=w1321:errorcluster)  [unwired: 13 in]
            n349 = call "Control_DAQ_Loop.vi"("Command (DAQ Control)"=DAQ_Control_Command."Shutdown", "Error In"=w1321) -> ("Error Out"=w1324:errorcluster)  [unwired: 13 in]
            n350 = call "Control_Cont_Send.vi"("Command (ERD Loop Control)"=GEA2_Control_Command."Shutdown", "Error In"=w1324) -> ("Error Out"=w1313:errorcluster)  [unwired: 13 in]
            n351 = call "Time Delay6"("error in (no error)"=w1313, "Delay Time (s)"=3.0) -> ("error out"=w1312:errorcluster)  [unwired: 9 in]
          }
          event "Tool Version": Value Change {
            n352 = event-data() -> ()  [unwired: 1 in, 6 out]
            n353 = property class="App"() -> ("App.Kind"=w1327:T55)  [unwired: 2 in, 2 out]
            n354 = case shown="\"Run Time System\"" w1327 {
              tunnel: ["invalid" ("File Version Info") w1330 w1335] -> w1328
              frame "invalid app kind", Default {
              }
              frame "Development System", "Student Edition".."Evaluation" {
                n355 = property class="App"() -> ("App.Version"=w1330:string)  [unwired: 2 in, 2 out]
              }
              frame "Run Time System" {
                n356 = property class="App"() -> ("App.Dir"=w1333:path, "App.Name"=w1334:string)  [unwired: 2 in, 2 out]
                n357 = Build Path(base path=w1333, name or relative path=w1334) -> (appended path=w1332:path)
                n358 = call <vilib>:"FileVersionInfo.vi"("Application Path in"=w1332) -> ("FileVersionInfo Out"=→"FileVersionInfo":T10, "File Version Info"=w1335:string)  [unwired: 7 in, 2 out]
              }
            }
            "LabView/Version Number" <- w1328
          }
        }
        n359 = call "Error_Control.vi"("Error In"=w654) -> ("Error Out"=w656:errorcluster)  [unwired: 14 in]
      }
      n360 = while "GEA2 Receive Message Loop" {
        shift-right: [w1339] -> w135
        shift-left: w62 -> [w1340]
        shift-right: [w1336] -> _
        shift-left: w47 -> [w1341]
        stop <- w1338 stop-if-true
        # "GEA2 Receive Message Loop"
        n361 = event shown="[2] <Data_Sent>: User Event" {
          selector: w1341 -> [w1352 _ w1375 w1383 w1402]
          dyn-events: [w1352 _ w1375 w1384 w1402] -> w1336
          timeout: _ -> [_ _ _ _ _]
          tunnel: w1340 -> [w1349 w1364 w1367 w1399 w1404]
          tunnel: [w1345 w1364 w1366 w1385 w1404] -> w1337
          tunnel: [FALSE TRUE FALSE _ TRUE] -> w1338
          event User Event {
            # "Added subscription Ack"
            n362 = event-data() -> ("Source"=w1354:u8, "Destination"=w1351:u8, "Command"=w1350:u8, "Message"=w1343:string)  [unwired: 1 in]
            n363 = Bundle By Name(cluster=T9 {"Source"=0, "Destination"=0, "Command"=0, "Message"=""} ("GEA2 Data In"), "Source"=w1354, "Destination"=w1351, "Command"=w1350, "Message"=w1343) -> (w1344:T9)
            n364 = call "GEA2 Log Filter.vi"("Filter Data"="Filter Data", "GEA2 Msg"=w1344, "Cmd to Filter"="Ignore this CMD", "error in (no error)"=w1349) -> ("error out"=w1346:errorcluster)  [unwired: 11 in]
            n365 = property on="Program Ind" class="Bool (strict)"() -> ("Value"=w1342:bool)  [unwired: 2 in, 2 out]
            n366 = case shown="False" w1342 {
              tunnel: w1346 -> [w1361 w1362]
              tunnel: [w1359 w1362] -> w1345
              tunnel: w1344 -> [w1357 _]
              frame False {
                n367 = call "FGV_GEA2_Ref.vi"("Action"=enum16{"Set Ref", "Get Ref"}."Get Ref", "Error In"=w1361) -> ("GEA2 Reference Out"=w1358:refnum<k24>, "Error Out"=w1360:errorcluster)  [unwired: 12 in]
                n368 = call "ACK Subscriptions Publications.vi"("GEA2 Reference In"=w1358, "GEA2 Msg"=w1357, "error in (no error)"=w1360) -> ("error out"=w1359:errorcluster)  [unwired: 11 in, 1 out]
              }
              frame True {
              }
            }
          }
          event User Event {
            n369 = event-data() -> ()  [unwired: 1 in, 7 out]
          }
          event User Event {
            # "This will update the UI with all data sent across the bus via a button Press"
            n370 = event-data() -> ("Source"=w1377:u8, "Destination"=w1374:u8, "Command"=w1373:u8, "Message"=w1372:string)  [unwired: 1 in]
            n371 = Bundle By Name(cluster=T9 {"Source"=0, "Destination"=0, "Command"=0, "Message"=""} ("GEA2 Data In"), "Source"=w1377, "Destination"=w1374, "Command"=w1373, "Message"=w1372) -> (w1368:T9)
            n372 = property on="Program Ind" class="Bool (strict)"() -> ("Value"=w1365:bool)  [unwired: 2 in, 2 out]
            n373 = call "GEA2MessageFormatter.vi"("Prefix(Send/Recv)"="SEND", "GEA2 Data In"=w1368, "Error In"=w1367) -> ("Output String"=w1371:string, "Error Out"=w1369:errorcluster)  [unwired: 11 in]
            n374 = case shown="False" w1365 {
              tunnel: w1371 -> [w1381 _]
              tunnel: w1369 -> [w1380 w1382]
              tunnel: [w1379 w1382] -> w1366
              frame False {
                n375 = call "GExplorer_Queue_GEA2.vi"("Output String"=w1381, "error in (no error)"=w1380) -> ("error out"=w1379:errorcluster)  [unwired: 13 in]
              }
              frame True {
              }
            }
          }
          event "Board Index": Value Change {
            # "Stop old GEA2\nbus reference"
            # "Allow other references a chance\nto begin using new reference"
            # "Store new GEA2 bus reference"
            # "Update event registration\nand initialize new GEA2 bus"
            # "Get the previous GEA2\nbus ref, but don't stop it\nuntil we update the FGV\nwith the new GEA2 ref"
            n376 = event-data() -> ("NewVal"=w1396:u8)  [unwired: 1 in]
            n377 = property on="Board Index" class="DigNum (strict)"(error in=w1399, "DisabledEnum"=T41."Disabled and Grayed Out" ("Disabled")) -> (error out=w1400:errorcluster)  [unwired: 1 in, 1 out]
            n378 = call "FGV_GEA2_Ref.vi"("Action"=enum16{"Set Ref", "Get Ref"}."Get Ref", "Error In"=w1400) -> ("GEA2 Reference Out"=w1389:refnum<k24>, "Error Out"=w1397:errorcluster)  [unwired: 12 in]
            n379 = call "GEA2_Reregister.vi"("Event Registration Refnum"=w1383, "Board Index"=w1396, "Error In"=w1397) -> ("GEA2 Reference Out"=w1394:refnum<k24>, "Board ID"=w1395:string, "Event Registration Refnum 2"=w1384:refnum<event-registration>, "Error Out"=w1388:errorcluster)  [unwired: 9 in]
            n380 = local write "Board ID"(w1395) -> ()
            n381 = call "FGV_GEA2_Ref.vi"("GEA2 Reference In"=w1394, "Action"=enum16{"Set Ref", "Get Ref"}."Set Ref", "Error In"=w1388) -> ("Error Out"=w1391:errorcluster)  [unwired: 11 in, 1 out]
            n382 = call "Time Delay"("error in (no error)"=w1391, "Delay Time (s)"=5.0) -> ("error out"=w1390:errorcluster)  [unwired: 9 in]
            n383 = call "GEA2 Stop.vi"("GEA2 Reference In"=w1389, "Error In"=w1390) -> ("Error Out"=w1386:errorcluster)  [unwired: 13 in]
            n384 = property on="Board Index" class="DigNum (strict)"(error in=w1386, "DisabledEnum"=T41."Enabled" ("Disabled")) -> (error out=w1385:errorcluster)  [unwired: 1 in, 1 out]
          }
          event "Stop": Value Change {
            n385 = event-data() -> ()  [unwired: 1 in, 6 out]
          }
        }
        n386 = call "Error_Control.vi"("Error In"=w1337) -> ("Error Out"=w1339:errorcluster)  [unwired: 14 in]
      }
      n387 = while "Continuous Send Loop" {
        shift-right: [w148] -> _
        shift-left: Cont_Send_States."Run" ("State") -> [w147]
        tunnel: w82 -> [w149]
        tunnel: [w142] -> _
        shift-right: [w140] -> w85
        shift-left: w62 -> [w151]
        stop <- w150 stop-if-true
        # "Continuous Send Loop"
        n388 = Dequeue Element(queue=w149, timeout in ms (-1)=0, error in (no error)=w151) -> (queue out=w143:refnum<queue>, element=w136:T35, timed out?=w144:bool, error out=w139:errorcluster)
        n389 = Select(t=w147, s=w144, f=w136) -> (s? t:f=w146:T35)
        n390 = property on="GEA2 Send" class="Clust (strict)"() -> ("Value"=w138:T9)  [unwired: 2 in, 2 out]
        n391 = case shown="\"Run\", Default" w146 {
          selector: w146 -> [w155 w166]
          tunnel: w139 -> [w157 w168]
          tunnel: [w156 w168] -> w141
          tunnel: [_ TRUE] -> w150
          tunnel: [w155 w166] -> w148
          tunnel: w143 -> [w154 w165]
          tunnel: [w154 w165] -> w142
          tunnel: w138 -> [w153 _]
          frame "Run", Default {
            n392 = case shown="True" "Start Send" {
              tunnel: w157 -> [w158 w161]
              tunnel: [w158 w164] -> w156
              tunnel: w153 -> [_ w163]
              frame False {
              }
              frame True {
                n393 = call "FGV_GEA2_Ref.vi"("Action"=enum16{"Set Ref", "Get Ref"}."Get Ref", "Error In"=w161) -> ("GEA2 Reference Out"=w160:refnum<k24>, "Error Out"=w159:errorcluster)  [unwired: 12 in]
                n394 = call "GEA2 Send Message.vi"("GEA2 Reference In"=w160, "Input Data"=w163, "Error In"=w159) -> ("Error Out"=w164:errorcluster)  [unwired: 11 in, 1 out]
              }
            }
          }
          frame "Shutdown" {
          }
        }
        n395 = call "Error_Control.vi"("Error In"=w141) -> ("Error Out"=w140:errorcluster)  [unwired: 14 in]
        n396 = Wait (ms)(milliseconds to wait="Msg Rate (ms)") -> ()  [unwired: 1 out]
      }
      n397 = while "GEA2 Display Loop" {
        tunnel: w63 -> [w372]
        shift-right: [w369] -> _
        shift-left: "" -> [w375]
        shift-right: [w371] -> w119
        shift-left: w79 -> [w379]
        tunnel: w77 -> [w365]
        tunnel: [w363] -> w75
        stop <- w373 stop-if-true
        # "GEA2 Display Loop"
        n398 = Dequeue Element(queue=w372, error in (no error)=w379) -> (element=w378:T40, error out=w374:errorcluster)  [unwired: 1 in, 2 out]
        n399 = Unbundle By Name(w378) -> ("Data"=w376:variant, "State"=w377:enum16{"Add to Log", "Clear", "Shutdown"})
        n400 = case shown="\"Add to Log\", Default" w377 {
          tunnel: w376 -> [w390 _ _]
          tunnel: w375 -> [w393 w398 _]
          tunnel: [w392 w398 ""] -> w370
          tunnel: w374 -> [w391 w399 w403]
          tunnel: [w388 w399 w403] -> w366
          tunnel: [FALSE TRUE FALSE] -> w373
          tunnel: [w380 _ _] -> w364
          frame "Add to Log", Default {
            n401 = Variant To Data(error in=w391, type="", Variant=w390) -> (data=w382:string, error out=w388:errorcluster)
            n402 = String Subset(string=w382, offset (0)=22, length (rest)=7 ("length (rest)")) -> (substring=w383:string)
            n403 = Equal?(x="SEND E5", y=w383) -> (x = y?=w381:bool)
            n404 = case shown="False" w381 {
              tunnel: w393 -> [w396 w397]
              tunnel: [w395 w397] -> w392
              tunnel: w382 -> [w394 _]
              tunnel: [w394 _] -> w380
              frame False {
                n405 = Concatenate Strings(w394, w396) -> (w395:string)
              }
              frame True {
              }
            }
          }
          frame "Shutdown" {
          }
          frame "Clear" {
          }
        }
        "GEA2 Log" <- w370
        n406 = call "Write _To_TXT_File.vi"("refnum"=w365, "text"=w364, "error in"=w366) -> ("refnum out"=w363:refnum<file>, "error out"=w367:errorcluster)  [unwired: 10 in, 1 out]
        n407 = String Subset(string=w370, length (rest)="GEA2 Log Length") -> (substring=w369:string)  [unwired: 1 in]
        n408 = call "Error_Control.vi"("Error In"=w367) -> ("Error Out"=w371:errorcluster)  [unwired: 14 in]
      }
      n409 = while "DAQ Loop" {
        shift-right: [w438] -> w118
        shift-left: w62 -> [w436]
        shift-right: [w422] -> _
        shift-left: DAQ_States."Wait for Init" ("States") -> [w433]
        shift-right: [w423] -> _
        shift-left: "Wait for Init" ("Report Text") -> [w432]
        shift-right: [w421] -> _
        shift-left: _ -> [w414]
        shift-right: [w420] -> _
        shift-left: w66 -> [w419]
        shift-right: [w418] -> _
        shift-left: w66 -> [w417]
        shift-right: [w416] -> _
        shift-left: w66 -> [w415]
        tunnel: w65 -> [w406]
        i -> [w404]
        stop <- w429 stop-if-true
        # "NI 9401 \nMódulo Digital Bidireccionales"
        # "NI 9263 \nMódulo de Salida de Voltaje"
        # "NI 9481 \nModulo de cuatro relevadores"
        # "DAQ Loop"
        n410 = Dequeue Element(queue=w406, timeout in ms (-1)=0, error in (no error)=w436) -> (element=w434:T36, timed out?=w435:bool, error out=w413:errorcluster)  [unwired: 1 out]
        n411 = Wait (ms)(milliseconds to wait=u32 100) -> ()  [unwired: 1 out]
        n412 = Select(t=w433, s=w435, f=w434) -> (s? t:f=w431:T36)
        n413 = case shown="\"Verify Hardware\"" w431 {
          selector: w431 -> [_ _ _ _ _ _ w626]
          tunnel: [w443 w453 w470 w506 w560 w576 w611] -> w427
          tunnel: w415 -> [w452 w463 w478 _ w554 w596 w619]
          tunnel: [w452 w463 w478 w498 w552 _ _] -> w416
          tunnel: w417 -> [w451 w461 w479 _ w536 w584 w602]
          tunnel: [w451 w461 w479 w491 w535 _ _] -> w418
          tunnel: [w441 w462 w466 w492 w537 w586 w604] -> w425
          tunnel: [w442 w464 w467 w499 w558 w595 w618] -> w426
          tunnel: [w448 DAQ_States."Verify Hardware" ("States") w475 DAQ_States."Run" ("States") w561 DAQ_States."Wait for Init" ("States") w626] -> w422
          tunnel: [FALSE FALSE FALSE TRUE TRUE FALSE FALSE] -> w421
          tunnel: [_ _ _ _ _ FALSE TRUE] -> w429
          tunnel: [w440 w460 w465 w486 w533 w574 w624] -> w424
          tunnel: [w450 w459 w480 w485 w531 _ _] -> w420
          tunnel: w419 -> [w450 w459 w480 _ w532 w573 w625]
          tunnel: [w449 "Rename Devices" ("Report Text") w472 "Initialize" ("Report Text") "Running" ("Report Text") "Wait for Init" ("Report Text") "Exit" ("Report Text")] -> w423
          tunnel: w432 -> [w449 _ _ _ _ _ _]
          tunnel: "Turn On DAQ" -> [w444 _ _ _ w559 _ _]
          tunnel: w413 -> [w443 w454 w468 w506 w560 w593 w612]
          tunnel: w413 -> [w442 w464 w467 w500 w548 w597 w620]
          tunnel: w413 -> [w441 w462 w466 w493 w538 w585 w603]
          tunnel: w413 -> [w440 w460 w465 w490 w534 w575 w622]
          tunnel: w414 -> [_ _ _ _ _ _ w621]
          tunnel: [_ _ _ _ w529 _ _] -> w412
          tunnel: [_ _ _ _ w528 _ _] -> w411
          tunnel: [_ _ _ _ w526 _ _] -> w410
          tunnel: [_ _ _ _ w525 _ _] -> w409
          tunnel: [_ _ _ _ w524 _ _] -> w408
          tunnel: [_ _ _ _ w521 _ _] -> w407
          tunnel: [_ _ _ _ w520 _ _] -> w405
          tunnel: w404 -> [_ _ _ _ w519 _ _]
          frame "Wait for Init", Default {
            # "DIO"
            # "Relays"
            # "AO"
            n414 = Select(t=DAQ_States."Rename Devices", s=w444, f=DAQ_States."Wait for Init" ("States")) -> (s? t:f=w448:T36)
          }
          frame "Rename Devices" {
            # "DIO"
            # "Relays"
            # "AO"
            n415 = call "Rename DAQ Devices.vi"("cDAQ Name"="JL_SLB", "Error In"=w454) -> ("Error Out"=w453:errorcluster)  [unwired: 13 in]
          }
          frame "Verify Hardware" {
            # "DIO"
            # "Relays"
            # "AO"
            n416 = call "DeviceListCheck.vi"("Device List"=string[] ["9401_1", "9481_1", "9263_1"], "Error In"=w468) -> ("Devices Present?"=w469:bool, "Report Text"=w472:string, "Error Out"=w471:errorcluster)  [unwired: 11 in]
            n417 = case shown="False" w469 {
              selector: w469 -> [w482 _]
              tunnel: w471 -> [w483 w484]
              tunnel: [w481 w484] -> w470
              frame False {
                n418 = property on="Turn On DAQ" class="Bool (strict)"(error in=w483, "Value"=w482) -> (error out=w481:errorcluster)  [unwired: 1 in, 1 out]
              }
              frame True {
              }
            }
            n419 = Select(t=DAQ_States."Initialize" ("f"), s=w469, f=DAQ_States."Wait for Init") -> (s? t:f=w475:T36)
          }
          frame "Initialize" {
            w488 = 0 items=["one channel for each line", "one channel for all lines"] ("line grouping")
            w495 = 0.0  # minimum value
            w496 = 5.0  # maximum value
            w503 = 0 items=["one channel for each line", "one channel for all lines"] ("line grouping")
            # "DIO"
            # "Relays"
            # "AO"
            n420 = call-poly <vilib>:"DAQmx Create Virtual Channel.vi"("lines"=tag "9481_1/port0/line0:3", "name to assign"="Relays", "line grouping"=w503, "error in"=w500) -> ("task out"=w498:refnum<k21>, "error out"=w499:errorcluster)  [unwired: 10 in]
            n421 = call-poly <vilib>:"DAQmx Create Virtual Channel.vi"("maximum value"=w496, "minimum value"=w495, "physical channels"=tag "9263_1/ao0:2" ("lines"), "name to assign"="AO", "error in"=w493) -> ("task out"=w491:refnum<k21>, "error out"=w492:errorcluster)  [unwired: 9 in]
            n422 = call-poly <vilib>:"DAQmx Create Virtual Channel.vi"("lines"=tag "9401_1/port0/line0:5", "name to assign"="DIO", "line grouping"=w488, "error in"=w490) -> ("task out"=w485:refnum<k21>, "error out"=w486:errorcluster)  [unwired: 10 in]
          }
          frame "Run" {
            # "DIO"
            # "Relays"
            # "AO"
            n423 = call-poly <vilib>:"DAQmx Read.vi"("task/channels in"=w532, "error in"=w534) -> ("task out"=w531:refnum<k21>, "data"=w530:bool[], "error out"=w533:errorcluster)  [unwired: 11 in]
            n424 = property on="Drum" class="Bool (strict)"() -> ("Value"=w522:bool)  [unwired: 2 in, 2 out]
            n425 = call "Outlet Convert Temp to Volt.vi"("Model IN"="Model", "Outlet Temperature"="Outlet Therm (F)", "Error In"=w538) -> ("Outlet Voltage"=w510:dbl, "Error Out"=w545:errorcluster)  [unwired: 11 in]
            "Outlet Voltage" <- w510
            n426 = Select(t=w522, s="CentSWControlType", f="CentSWControl") -> (s? t:f=w521:bool)
            n427 = Not(x="Normal Temp V") -> (.not. x?=w511:bool)
            n428 = Index Array(array=w530) -> (element #1=w529:bool, element #2=w528:bool, element #3=w527:bool, element #4=w525:bool, element #5=w524:bool, element #6=w520:bool)  [unwired: 6 in]
            n429 = case shown="True" "CentSWControlType" {
              tunnel: [T41."Enabled" ("Disabled") T41."Disabled and Grayed Out" ("Disabled")] -> w551
              tunnel: [w568 w570] -> w549
              tunnel: w548 -> [w568 w570]
              frame False {
              }
              frame True {
              }
            }
            n430 = call "Inlet_Temp_To_Voltage.vi"("Model"=enum16{"Estar Centauro", "GFL"}."GFL", "Temperature"="Inlet Therm (F)", "Error In"=w545) -> ("Voltage"=w513:dbl, "Error Out"=w544:errorcluster)  [unwired: 11 in]
            "Inlet Voltage" <- w513
            n431 = case shown="True" w527 {
              tunnel: ["CCW" "CW"] -> w526
              frame False {
              }
              frame True {
              }
            }
            n432 = Select(t="Manual Inlet", s=w511, f=w513) -> (s? t:f=w514:dbl)
            n433 = property on="CentSWControl" class="Bool (strict)"(error in=w549, "DisabledEnum"=w551) -> (error out=w550:errorcluster)  [unwired: 1 in, 1 out]
            n434 = Select(t="Manual Outlet", s=w511, f=w510) -> (s? t:f=w516:dbl)
            n435 = call "Dither.vi"("Moisture (V) in"="Moisture (V)", "Dither"="Dither (V)", "Iteration Terminal"=w519, "Error In"=w544) -> ("Moisture (V)"=w540:dbl, "Error Out"=w543:errorcluster)  [unwired: 10 in]
            n436 = Select(t=DAQ_States."Run" ("States"), s=w559, f=DAQ_States."Shutdown" ("States")) -> (s? t:f=w561:T36)
            n437 = Build Array(w521, "Door Status", "AC Power", "Start Signal") -> (w553:bool[])
            n438 = Build Array(w516, w514, w540) -> (w546:dbl[])
            n439 = call-poly <vilib>:"DAQmx Write.vi"("task/channels in"=w554, "data"=w553, "error in"=w550) -> ("task out"=w552:refnum<k21>, "error out"=w558:errorcluster)  [unwired: 10 in, 1 out]
            n440 = call-poly <vilib>:"DAQmx Write.vi"("task/channels in"=w536, "data"=w546, "error in"=w543) -> ("task out"=w535:refnum<k21>, "error out"=w537:errorcluster)  [unwired: 10 in, 1 out]
          }
          frame "Shutdown" {
            w591 = 0.0
            # "This Value is Gets You within 20 \nof Thershold of 2400         ===>"
            # "DIO"
            # "Relays"
            # "AO"
            n441 = property on="Turn On DAQ" class="Bool (strict)"(error in=w593, "Value"=FALSE ("Turn On DAQ")) -> (error out=w579:errorcluster)  [unwired: 1 in, 1 out]
            n442 = property on="CentSWControlType" class="Bool (strict)"(error in=w579, "Value"=TRUE ("CentSWControlType")) -> (error out=w577:errorcluster)  [unwired: 1 in, 1 out]
            n443 = Build Array(w591, w591, w591) -> (w592:dbl[])
            n444 = call-poly <vilib>:"DAQmx Write.vi"("task/channels in"=w584, "data"=w592, "error in"=w585) -> ("task out"=w572:refnum<k21>, "error out"=w590:errorcluster)  [unwired: 10 in, 1 out]
            n445 = call <vilib>:"DAQmx Clear Task.vi"("task in"=w573, "error in"=w575) -> ("error out"=w574:errorcluster)  [unwired: 13 in]
            n446 = call <vilib>:"DAQmx Clear Task.vi"("task in"=w596, "error in"=w597) -> ("error out"=w595:errorcluster)  [unwired: 13 in]
            n447 = call <vilib>:"DAQmx Clear Task.vi"("task in"=w572, "error in"=w590) -> ("error out"=w589:errorcluster)  [unwired: 13 in]
            n448 = property on="Outlet Therm (F)" class="Knob (strict)"(error in=w589, "Value"=75.0 ("Outlet Therm (F)")) -> (error out=w588:errorcluster)  [unwired: 1 in, 1 out]
            n449 = property on="CentSWControl" class="Bool (strict)"(error in=w577, "DisabledEnum"=T41."Disabled and Grayed Out" ("Disabled")) -> (error out=w576:errorcluster)  [unwired: 1 in, 1 out]
            n450 = property on="Inlet Therm (F)" class="Knob (strict)"(error in=w588, "Value"=75.0 ("Inlet Therm (F)")) -> (error out=w587:errorcluster)  [unwired: 1 in, 1 out]
            n451 = property on="Moisture (V)" class="Slide (strict)"(error in=w587, "Value"=1.84511 ("Moisture (V)")) -> (error out=w586:errorcluster)  [unwired: 1 in, 1 out]
          }
          frame "Exit" {
            # "This Value is Gets You within 20 \nof Thershold of 2400         ===>"
            n452 = case shown="True" w621 {
              tunnel: w619 -> [_ w644]
              tunnel: [w629 w643] -> w605
              tunnel: [w631 w642] -> w618
              tunnel: w625 -> [_ w641]
              tunnel: [w630 w640] -> w624
              tunnel: w620 -> [w631 w639]
              tunnel: w622 -> [w630 w638]
              tunnel: w603 -> [w629 w633]
              tunnel: w602 -> [_ w632]
              frame False {
              }
              frame True {
                w636 = 0.0
                # "DIO"
                # "Relays"
                # "AO"
                n453 = Build Array(w636, w636, w636) -> (w637:dbl[])
                n454 = call-poly <vilib>:"DAQmx Write.vi"("task/channels in"=w632, "data"=w637, "error in"=w633) -> ("task out"=w635:refnum<k21>, "error out"=w634:errorcluster)  [unwired: 10 in, 1 out]
                n455 = call <vilib>:"DAQmx Clear Task.vi"("task in"=w644, "error in"=w639) -> ("error out"=w642:errorcluster)  [unwired: 13 in]
                n456 = call <vilib>:"DAQmx Clear Task.vi"("task in"=w635, "error in"=w634) -> ("error out"=w643:errorcluster)  [unwired: 13 in]
                n457 = call <vilib>:"DAQmx Clear Task.vi"("task in"=w641, "error in"=w638) -> ("error out"=w640:errorcluster)  [unwired: 13 in]
              }
            }
            n458 = property on="Turn On DAQ" class="Bool (strict)"(error in=w612, "Value"=FALSE ("Turn On DAQ")) -> (error out=w615:errorcluster)  [unwired: 1 in, 1 out]
            n459 = property on="CentSWControlType" class="Bool (strict)"(error in=w615, "Value"=TRUE ("CentSWControlType")) -> (error out=w613:errorcluster)  [unwired: 1 in, 1 out]
            n460 = property on="Outlet Therm (F)" class="Knob (strict)"(error in=w605, "Value"=75.0 ("Outlet Therm (F)")) -> (error out=w610:errorcluster)  [unwired: 1 in, 1 out]
            n461 = property on="CentSWControl" class="Bool (strict)"(error in=w613, "DisabledEnum"=T41."Disabled and Grayed Out" ("Disabled")) -> (error out=w611:errorcluster)  [unwired: 1 in, 1 out]
            n462 = property on="Inlet Therm (F)" class="Knob (strict)"(error in=w610, "Value"=75.0 ("Inlet Therm (F)")) -> (error out=w609:errorcluster)  [unwired: 1 in, 1 out]
            n463 = property on="Moisture (V)" class="Slide (strict)"(error in=w609, "Value"=1.84511 ("Moisture (V)")) -> (error out=w604:errorcluster)  [unwired: 1 in, 1 out]
          }
        }
        "DAQ Status" <- w423
        "DAQ On?" <- w421
        "Steam" <- w412
        "Drum" <- w411
        "Drum Direction" <- w410
        "Inner/Gas Coil" <- w409
        "Outer Coil" <- w408
        "Drum Light" <- w405
        "Centrifugal Switch" <- w407
        n464 = Merge Errors(w427, w426, w425, w424) -> (w428:errorcluster)
        n465 = call "Error_Control.vi"("Error In"=w428) -> ("Error Out"=w438:errorcluster)  [unwired: 14 in]
      }
      n466 = Close File(refnum=w75, error in=w119) -> (error out=w76:errorcluster)  [unwired: 1 out]
      n467 = call "GEA2 Stop.vi"("GEA2 Reference In"=w133, "Error In"=w134) -> ("Error Out"=w128:errorcluster)  [unwired: 13 in]
      n468 = Close File(refnum=w89, error in=w91) -> (error out=w90:errorcluster)  [unwired: 1 out]
      n469 = Merge Errors(w90, w76, w85, w135, w128, w118) -> (w116:errorcluster)
      n470 = Obtain Queue(name (unnamed)="Continuous Send", element data type=Cont_Send_States."Run" ("State")) -> (queue out=w88:refnum<queue>, error out=w87:errorcluster)  [unwired: 3 in, 1 out]
      n471 = Obtain Queue(name (unnamed)="ERD Loop", element data type=T37 {"Data"=variant, "State"=enum."Read ERDs"} ("Data"), error in (no error)=w116) -> (queue out=w125:refnum<queue>, error out=w124:errorcluster)  [unwired: 2 in, 1 out]
      n472 = Obtain Queue(name (unnamed)="GEA2", element data type=T40 {"Data"=variant, "State"=enum."Add to Log"} ("Data"), error in (no error)=w116) -> (queue out=w132:refnum<queue>, error out=w131:errorcluster)  [unwired: 2 in, 1 out]
      n473 = Obtain Queue(name (unnamed)="DAQ", element data type=DAQ_States."Wait for Init" ("States"), error in (no error)=w116) -> (queue out=w120:refnum<queue>, error out=w121:errorcluster)  [unwired: 2 in, 1 out]
      n474 = Release Queue(queue=w88, error in (no error)=w87) -> (error out=w86:errorcluster)  [unwired: 1 in, 2 out]
      n475 = Release Queue(queue=w125, error in (no error)=w124) -> (error out=w113:errorcluster)  [unwired: 1 in, 2 out]
      n476 = Release Queue(queue=w132, error in (no error)=w131) -> (error out=w114:errorcluster)  [unwired: 1 in, 2 out]
      n477 = Release Queue(queue=w120, error in (no error)=w121) -> (error out=w115:errorcluster)  [unwired: 1 in, 2 out]
      n478 = Merge Errors(w86, w113, w114, w115) -> (w112:errorcluster)
      n479 = call "Error_Control.vi"("Command (Handle Errors)"=Error_Command."Report Errors", "Error In"=w112) -> ("Error Out"=w111:errorcluster)  [unwired: 13 in]
    }
    frame Error {
    }
  }
  n480 = call <vilib>:"Simple Error Handler.vi"("error in (no error)"=w31) -> ("error out"=→"Error Out":errorcluster)  [unwired: 4 in, 4 out]
